vi "UHR-Fleezers Control (fpga) - avogadro 4 - laser switching test.vi"() -> ()   [LabVIEW 2014]
doc: "UHR-Fleezers Instrument Control Code (fpga)"
uses:
  <vilib>/Platform/TimedLoop/XDataNode/timing_clust.ctl
  <vilib>/Platform/TimedLoop/XDataNode/nitl_modes.ctl
  <vilib>/Platform/TimedLoop/XDataNode/wakeup.ctl
  <vilib>/rvi/Emulation/niFpgaGetClockAttributes.vi
  <vilib>/rvi/Emulation/niFpgaSctlEmulationGetInTimedLoop.vi
  <vilib>/rvi/Emulation/niFpgaEmulationReportErrorSimple.vi
  <vilib>/rvi/Emulation/niFpgaProcessEmulError.vi
  <vilib>/rvi/eio/common/nirviEmuTemplateMethod_errors.vi
  <vilib>/rvi/interface/RandomDataEmulation/niFpgaRandomDataHandleErrors.vi
  <vilib>/rvi/Emulation/niFpgaCriticalErrorInLSC.vi
  <vilib>/rvi/Emulation/niFpgaEmulationIsFPGAContextNoSignature.vi
  <vilib>/rvi/errors/niFpgaSetErrorForExecOnDevCompSimple.vi
  <vilib>/rvi/eio/common/nirviEmuReportErrorAndStop.vi
  <vilib>/rvi/DataTransferAndStorage/Container/Common/niFpgaContainerGetUniqueNameForEmu.vi
  <vilib>/rvi/FIFO/Fifo_Resource/nirvififoEmulationSetSize.vi
  <vilib>/rvi/FIFO/Fifo_Resource/nirviFifoEmulationQueueMgr.vi
  <instcachedir>/0/nirviFifoEmulationQueueMgr_E5CAEC123FF24DC58D834DCA3CDAA9B5.lvgen/nirviFifoEmulationQueueMgr_E5CAEC123FF24DC58D834DCA3CDAA9B5_001.vi
  <vilib>/rvi/FIFO/Fifo_Resource/nirvififoEmulationDetermineInputValidOut.vi
  <vilib>/rvi/FIFO/Fifo_Resource/nirvififoEmulationCreateLock.vi
  <vilib>/rvi/FIFO/Fifo_Resource/nirvififoEmulationObtainLock.vi
  <vilib>/rvi/FIFO/Fifo_Resource/nirvififoEmulationReleaseLock.vi
  <vilib>/rvi/occurrence/nirviWaitOnOccurrenceBase.vi
  <vilib>/rvi/errors/nirviReportUnexpectedCaseInternalError.vi
  <vilib>/rvi/errors/nirviReportUnexpectedCaseInternalError (U32).vi
  <vilib>/rvi/DataTransferAndStorage/Container/Common/niFpgaContainerExecOnDevCompGetState.vi
  <vilib>/Utility/error.llb/Clear Errors.vi
  <vilib>/rvi/Memory/Memory_Emulation/niFpgaMemoryEmulationCacheClearOnFirstRun.vi
  <vilib>/rvi/Memory/Memory_Emulation/nirvimemoryEmulationManagerCache_MakeExclusive.vi
  <vilib>/rvi/Memory/Memory_Emulation/niFpgaMemoryEmulationValidateCache.vi
  <vilib>/rvi/Memory/Memory_Emulation/nirvimemoryEmulationManagerCache_InsertValue.vi
  <vilib>/rvi/Memory/Memory_Emulation/nirvimemoryEmulationManagerCache_ReleaseExclusive.vi
  <vilib>/rvi/Memory/Memory_Emulation/nirvimemoryEmulationManagerCache_GetValue.vi
  <vilib>/rvi/Memory/Memory_Emulation/nirvimemoryEmulationManagerCache_SetValue.vi
  <vilib>/rvi/Emulation/niFpgaSctlEmulationResourceMgr.vi
  <vilib>/eio/EIONode/EIONode.xnode
  <vilib>/eio/EIOMethodNode/EIOMethodNode.xnode
  <vilib>/rvi/DataTransferAndStorage/Container/XNode/niFpgaContainer.xnode
  <vilib>/rvi/interface/RandomDataEmulation/nirviRandomDataFpgaReadWriteTemplate.vi
  <vilib>/rvi/FIFO/Fifo_Resource/nirvififoEmulationWrite.vi
  <vilib>/rvi/FIFO/Fifo_Resource/niFpgaFifoEmulationRefIn.vi
  <vilib>/rvi/Memory/Memory_Emulation/niFpgaMemoryEmulationRefIn.vi
  <vilib>/addons/control/pid/fpga.llb/XNode/niFpgaPID.xnode
  <vilib>/Platform/TimedLoop/XDataNode/XDataNode.xnode
  <vilib>/rvi/FIFO/Fifo_Resource/nirvififoEmulationRead.vi
  <vilib>/Platform/TimedLoop/XDataNode/XDNodeRunTimeDep.lvlib
panel:
  in  "BD 1 Delay (ticks)":u8
  out "lifetime (ticks)":u16
  in  "Lifetime to FIFO":bool
  in  "Tab Control":T1(tab)=enum."MCL trap control"
  in  "Set 3":bool
  in  "Set 2":bool=TRUE
  in  "Set 1":bool=TRUE
  in  "Trap Pos to FIFO":bool
  in  "N of AI1 Int Acq Sets":i16=2 min=1 max=3 step=1
  out "AI Late Counter":u8
  in  "ai count":u16=400
  in  "+ phase":bool
  in  "Phase count adjustment":i16
  out "Relative phase":i16
  in  "AI to FIFO":bool
  out "BD1 Frequency Out 1":u64
  out "BD1 Frequency Out 2":u64
  out "Trap Pos FIFO Timeout":u16
  out "Trap AI FIFO Timeout":u16
  in  "Trap FIFO Set Timeout":i32
  in  "Tab Control 2":T2(tab)
  in  "Multiple trap 3 position offset \nfile":bool
  in  "Piezo offset Y points":u64
  in  "Piezo offset X points":u64
  in  "Piezo offset Xmin":u64
  in  "Piezo Offset Ymin":u64
  in  "Piezo Offset Increment":u64
  out "BD1 amplitude 1 out":u16
  out "BD1 amplitude 2 out":u16
  in  "FB output range":cluster{"output low":i16, "output high":i16}={"output low"=0, "output high"=3000}
  in  "FB Gains":T3={"proportional gain (Kc)"=10, "integral gain (Kc*Ts/Ti)"=5, "derivative gain (Kc*Td/Ts)"=0}
  in  "RF synth green feedback max":i16=4000
  in  "RD":bool=TRUE
  in  "Swap F1 and F2":bool
  in  "Cont. Scan":bool
  in  "Abort scan":bool
  in  "Cycles per step":u64
  in  "Scan BD":bool
  in  "Number of scans":u16
  in  "Scan steps":u64
  in  "Scan freq.  increment":i64
  out "Scanning":bool
  in  "Start scan":bool
  in  "OSK Bd 1":bool
  in  "Reset Bd 1":bool
  in  "PMODE":bool=TRUE
  in  "Number Interlace Cycles":u8=2 min=1 max=3
  in  "Interlace Off Parameters":u8=1 min=1 max=3
  in  "Interlace ON/OFF":bool
  out "DIO Relative phase":i16
  in  "Phase count adjustment (DIO)":i16
  in  "+ phase (DIO)":bool
  out "DIO Late Counter":u8
  in  "DIO count 1 (ticks)":u16=400
  in  "DIO count 2 (ticks)":u16=400
  in  "DIO count 3 (ticks)":u16=400
  out "AI2 Y Sum Set 2":i16
  out "AI2 Y Sum Set 1":i16
  in  "FB Setpoint Set 1":i16 min=0 step=1
  in  "FB Reset Set 1":bool
  in  "FB On/Off Set 1":bool
  in  "FB Reset Set 2":bool
  in  "FB On/Off Set 2":bool
  in  "FB Setpoint Set 2":i16 min=0 step=1
  out "Scan I":u64
  in  "Amp switch delay":u8=5
  in  "RF synth bd controls green":bool
  in  "Phase Trap 2":fxp<+,14,14>
  in  "Phase Trap 1":fxp<+,14,14>
  in  "Phase offset method":u8
  in  "BD 2 Amplitude 1":u16
  in  "BD 1 Amplitude 1":u16
  in  "BD 2 Frequency 1":u64
  in  "BD 1 Frequency 1":u64
  in  "BD 2 Amplitude 2":u16
  in  "BD 1 Amplitude 2":u16
  in  "BD 2 Frequency 2":u64
  in  "BD 1 Frequency 2":u64
  in  "BD 2 Amplitude 3":u16
  in  "BD 1 Amplitude 3":u16
  in  "BD 2 Frequency 3":u64
  in  "BD 1 Frequency 3":u64
  in  "BD 2 Delay (Ticks)":u8 caption="Count(Ticks)"
  in  "Next trap write delay (ticks)":u8 caption="Count(Ticks)"
  out "Random phase generated":fxp<+,14,14>
  in  "RF phase reset before cycles":bool
  in  "Trap 1 osc enable":bool
  in  "N trap osc periods":i16
  in  "Trap osc period (pts)":i16
  in  "Osc traps":bool
  in  "Initiate trap osc":bool
  in  "Ready Write":bool
  in  "Data":i64
  in  "Address 2":u32
  in  "Osc trap cont.":bool
  in  "Trap 2 osc enable":bool
  out "Piezo X out":i16
  out "Piezo Y out":i16
  in  "Piezo Trap ON/Off (AO3)":i16
  in  "Piezo Trap X (AO5)":i16
  in  "Piezo Trap Y (AO4)":i16
  in  "FB Min frequency":u64
  in  "FB Max Frequency":u64
  in  "Dynamic Force FB (Ronen)":bool
  in  "Trap pos. FB Range":T4={"FB2 output low"=-1.0, "FB2 output high"=0.999969482421875}
  in  "Trap Pos. FB Gains":T5={"proportional gain (Kc)"=0.999969482421875, "integral gain (Kc*Ts/Ti)"=0.999969482421875, "derivative gain (Kc*Td/Ts)"=0.0}
  in  "B factor":fxp<+/-,32,16>
  in  "Negate Diff?":bool
  in  "Diff FB Measurement?":bool
  in  "FB Trig Integrate":u32=1
  out "TTrig?":bool
  in  "TTrig Negate Pos":bool=TRUE
  out "Trap Pos FB Int Signal":fxp<+/-,24,9> format="%.18g"
  out "Trap Pos FB Int-Norm Signal":fxp<+/-,16,1> format="%.16g"
  in  "FPGA TTrig Thresh":i64
  in  "FPGA Trap Trig":bool
  out "Trap Pos FB Action":i64
  in  "Trap Pos. FB Offset Factor":i64
  in  "Trap Pos. FB Mult Factor":i64=2
  in  "Trap Pos. FB Reset":bool
  in  "Trap Pos FB Monitor T1 or T2":bool
  in  "AI1 X Scale":u16
  in  "Trap Pos FB Int Count":u16=100
  in  "Trap Pos FB Negate Action":bool
  out "AI1 X Set 2":fxp<+/-,16,1>
  out "AI1 X Set 1":fxp<+/-,16,1>
  in  "Trap Pos. FB SP":fxp<+/-,16,1>
  in  "Force feedback":bool
  out "TTrig Sig":i64
  out "TTrig Fin Thresh":i64
  in  "ScanTrap 3 or Fl-laser":bool
  in  "1D or 2D Scan?":bool
  in  "Abort scan (MCL)":bool
  in  "MCL Scan Axis":bool
  in  "Cont. Scan (MCL)":bool
  out "Scan I (MCL)":u64
  in  "Number of scans (MCL)":u16
  out "Scanning MCL":bool
  in  "Scan steps (MCL)":u64
  in  "Cycles per step (MCL)":u64
  in  "Scan freq.  increment (MCL)":i16
  in  "Start scan (MCL)":bool
  in  "AO2 (X)":i16
  in  "AO1 (Y)":i16
  out "MCL Late Counter":u8
  in  "MCL count":u32=800
  out "MCL Relative Phase":i16
  in  "Phase count adjustment (MCL)":i16
  in  "+ phase (MCL)":bool
  in  "Lifetime events to read blue":u16=100
  in  "Lifetime read blue fifo":bool
  out "lifetime events in fifo":u16
  out "APD2 int gate":bool
  out "APD3 out state":bool
  in  "APD Gate Operating Mode":u8 max=2 step=1
  in  "Invert APD Gate":bool
  in  "APD Gate OFF Count":u16=100
  in  "APD Gate ON Count":u16=300
  out "APD 1 Gate Late Counter":u8
  out "APD 1 Gate Relative Phase":i16
  in  "Phase count adjustment (APD 1 Gate)":i16
  in  "+ phase (APD 1 Gate)":bool
  out "APD 2 Counts 0":u32
  out "APD 2 Counts 1":u32
  out "APD 1 Counts 0":u32
  out "APD 1 Counts 1":u32
  out "APD1 out state":bool
  in  "APD AO scale factor":i16=1
  in  "APD to FIFO":bool
  in  "APD Acq Rate Count":u32=20000000
  out "APD Acq Late Counter":u8
  out "APD Acq Relative Phase":i16
  in  "Phase Count Adjustment (APD Acq)":i16
  in  "+ phase (APD Acq)":bool
  in  "Phase count adjustment (APD 2 Gate)":i16
  out "APD 2 Gate Late Counter":u8
  out "APD 2 Gate Relative Phase":i16
  in  "+ phase (APD 2 Gate)":bool
  out "APD2 out state":bool
  out "APD 3 Counts 0":u32
  out "APD 3 Counts 1":u32
  out "APD 3 Gate Late Counter":u8
  in  "Phase count adjustment (APD 3 Gate)":i16
  out "APD 3 Gate Relative Phase":i16
  in  "+ phase (APD 3 Gate)":bool
  out "APD1 int gate":bool
  out "APD3 int gate":bool
  in  "Lifetime timeout APD1":u16=200
  in  "Laser choice 2":u8=100
  in  "Laser choice 1":u8=100
  in  "Laser choice 0":u8=100
  in  "FL interlace OFF count 2":u16=100
  in  "FL interlace OFF count 1":u16=100
  in  "FL interlace ON count 2":u16=300
  in  "Fl interlace ON count 1":u16=300
  in  "D3 2":i16
  in  "I3 2":i16=5
  in  "P3 2":i16=10
  in  "Green FB Setpoint 2":i16=250 min=0 step=1
  in  "Green FB Reset 2":bool
  in  "D3":i16
  in  "I3":i16=5
  in  "P3":i16=10
  in  "Green Filter Flipper":bool
  in  "Green FB Count":u16=1200
  out "Green Late Counter":u8
  out "Green FB Relative Phase":i16
  in  "Phase count adjustment (Green FB)":i16=10
  in  "+ phase (Green FB)":bool
  out "Green FB Sum":i16
  in  "Green int current ON count adj":u16=150
  in  "Current Out":u16=30000
  in  "Green FB On/Off":bool
  in  "Green FB Setpoint":i16=250 min=0 step=1
  in  "Green FB Reset":bool
  in  "Operating Mode 2":u8=2 max=2 step=1
  in  "Invert GI 2":bool
  in  "Green interlace OFF count 2":u16=900
  in  "Green interlace ON count 2":u16=300
  out "GI Late Counter 2":u8
  out "GI Relative phase 2":i16
  in  "Phase count adjustment (GI) 2":i16=20
  in  "+ phase (GI) 2":bool
  in  "FL interlace OFF count 0":u16=100
  out "GI Relative phase":i16
  in  "Phase count adjustment (GI)":i16
  in  "+ phase (GI)":bool
  in  "FL interlace ON count 0":u16=300
  out "GI Late Counter":u8
  in  "Invert GI":bool
  in  "Operating Mode":u8 max=2 step=1
  out "green FB running":bool
  in  "+ phase (RI)":bool
  out "RI Relative phase":i16
  out "RI Late Counter":u8
  in  "Red interlace ON count":u16=300
  in  "Red interlace OFF count":u16=100
  in  "Invert RI":bool
  in  "Red Laser Operating Mode":u8 max=2 step=1
  in  "Phase count adjustment (RI)":i16
  out "Red FB Intensity":i16
  in  "RI Current Out":u16=30000
  in  "Red FB On/Off":bool
  in  "D4":i16
  in  "I4":i16=5
  in  "P4":i16=10
  in  "Red FB Setpoint":i16=250 min=0 step=1
  in  "Red FB Reset":bool
  in  "RI Operating Mode 2":u8=2 max=2 step=1
  in  "Invert RI 2":bool
  in  "Phase count adjustment (BI AO)":i16=20
  in  "Blue current ON count adj (AO)":u16=150
  in  "BI Current Out":i16=30000
  in  "Blue FB On/Off":bool
  in  "D5":i16
  in  "I5":i16=5
  in  "P5":i16=10
  in  "Blue FB Setpoint":i16=250 min=0 step=1
  in  "Blue FB Reset":bool
  in  "BI Operating Mode (AO)":u8=2 max=2 step=1
  in  "Invert BI (AO)":bool
  in  "Blue OFF count (AO)":u16=900
  in  "Blue ON count (AO)":u16=300
  out "BI Late Counter (AO)":u8
  out "BI Relative phase (AO)":i16
  in  "+ phase (BI AO)":bool
  in  "Phase count adjustment (BI D)":i16
  in  "Blue Laser Operating Mode (D)":u8 max=2 step=1
  in  "Invert BI (D)":bool
  in  "Blue interlace OFF count (D)":u16=100
  in  "Blue interlace ON count (D)":u16=300
  out "Blue Late Counter (D)":u8
  out "BI Relative phase (D)":i16
  in  "+ phase (BI D)":bool
  out "Blue Intensity":i16
  in  "Invert EMCCD Gate":bool
  in  "EMCCD Gate ON count":u16=300
  in  "EMCCD Gate OFF count":u16=100
  out "EMCCD Late counter":u8
  out "EMCCD relative phase":i16
  in  "+ phase (EMCCD Gate)":bool
  in  "EMCCD Gate Operating Mode":u8 max=2 step=1
  in  "Phase Count Adjustment EMCCD Gate":i16
  # "Raster Scan AOD"
  # "1 (X)"
  # "2 (Y)"
  # "IR Intensity Feedback (RF BD 1)"
  # "FB Gains Set 1"
  # "FB output range 1"
  # "IR Intensity Feedback (RF BD 2) -\nonly when using BD 2 for green laser AOM (not trap Y)"
  # "Keep below 4096 (12 bits) to stay within range of RF board. Going over doesn't saturate, it truncates higher bits."
  # "RF phase offset control"
  # "Methods are:\n0 - Default, do nothing at all (no phase offset writes)\n1 - Manual phase adjustment\n2 - Cycle the phase adjustment using the input phase numbers as increment values for each cycle"
  # "False is usual, True is external loop method"
  # "Parameters if using the external RF switching loop"
  # "Parameters if using the usual internal RF switching method"
  # "FB Triggering Excitation Laser"
  # "Trap Pos. FB Gains"
  # "Trap Pos. FB Range"
  # "AO1 (Y)"
  # "2D"
  # "Trap 3"
  # "1D"
  # "AO2 (X)"
  # "Fl Laser"
  # "APD AO for aligning"
  # "Detection Loop"
  # "Green fluorescent laser digital gate interlacing loop"
  # "0 Forced ON\n1 Forced OFF\n2 Interlacing"
  # "ALEX settings:"
  # "Controls for usual IA ME controls green AOM"
  # "Controls for RF synth board controls green AOM"
  # "Green FB Gains"
  # "Red fluorescent laser digital gate interlacing loop"
  # "Detection Loop"
  # "0 Forced ON\n1 Forced OFF\n2 Interlacing"
  # "Analog/FB Control Loop\n(Disabled)"
  # "Digital Control Loop"
  # "Blue laser intensity reading"
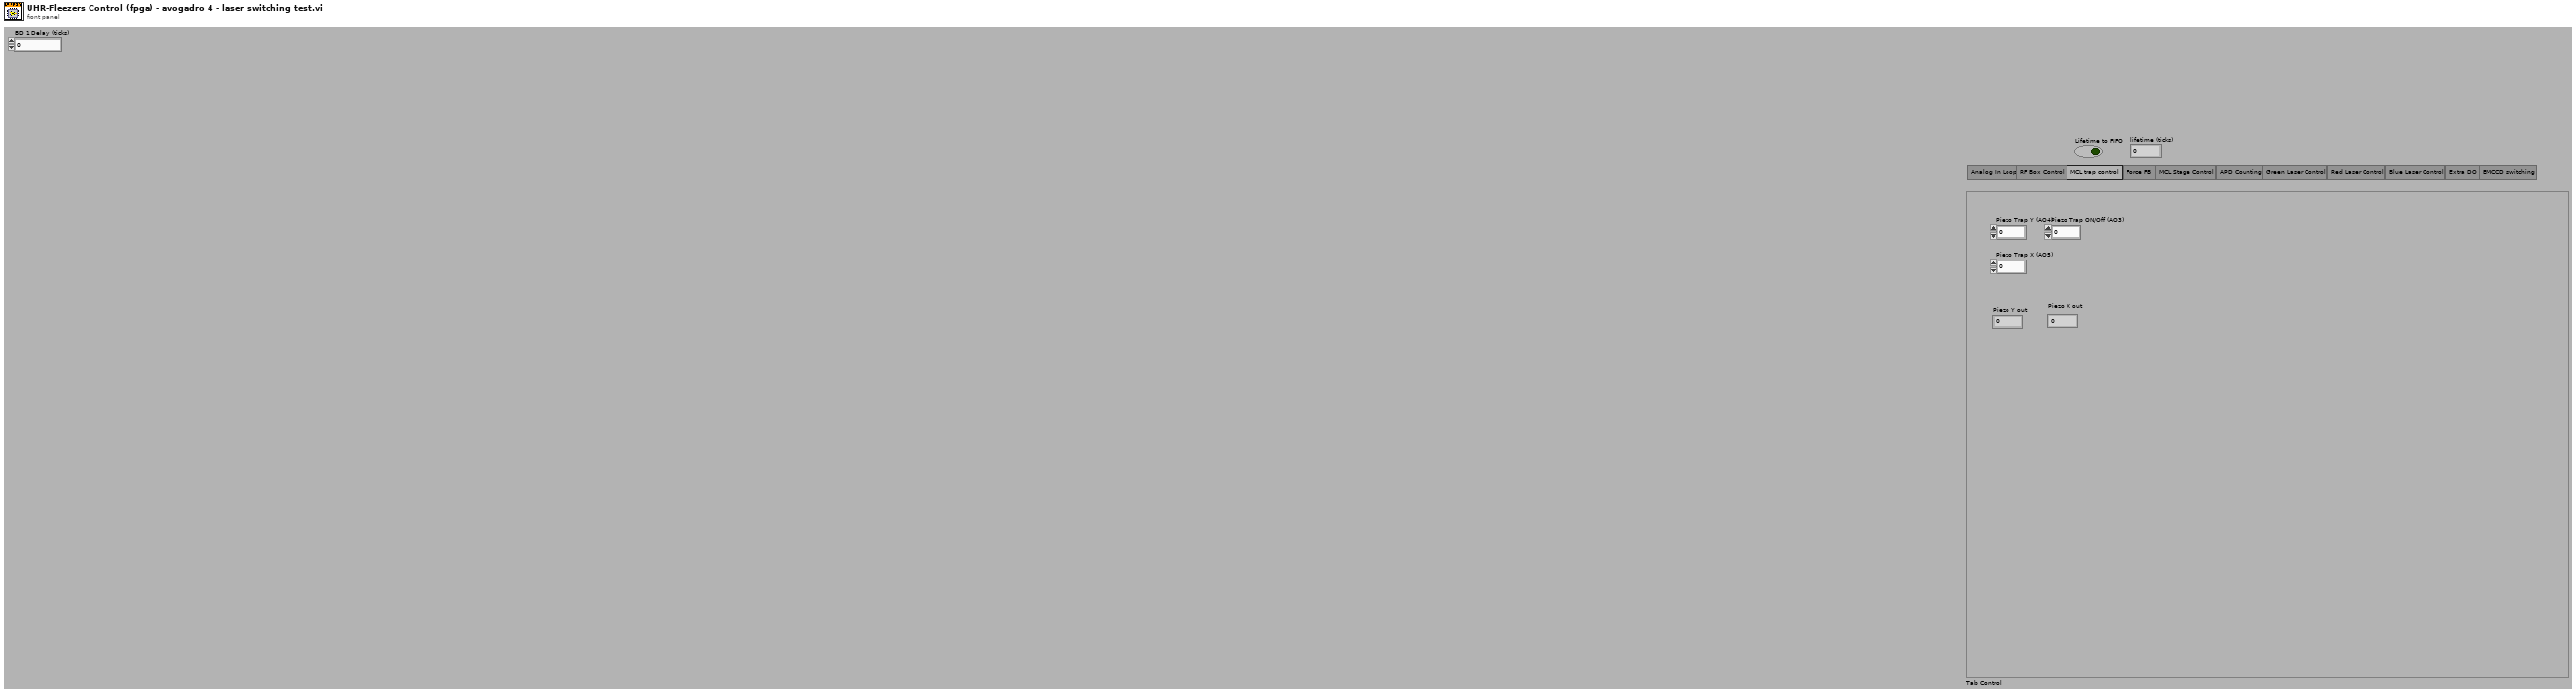
[diagram p1: front panel]
types:
  T1 = enum32{"Analog In Loop", "RF Box Control", "MCL trap control", "Force FB", "MCL Stage Control", "APD Counting", "Green Laser Control", "Red Laser Control", "Blue Laser Control", "Extra DO", "EMCCD switching"}
  T2 = enum32{"Controls", "Interlacing Frequency and Amplitude Values", "Oscillate trap from memory"}
  T3 = cluster{"proportional gain (Kc)":i16, "integral gain (Kc*Ts/Ti)":i16, "derivative gain (Kc*Td/Ts)":i16}
  T4 = cluster{"FB2 output low":fxp<+/-,16,1>, "FB2 output high":fxp<+/-,16,1>}
  T5 = cluster{"proportional gain (Kc)":fxp<+/-,16,1>, "integral gain (Kc*Ts/Ti)":fxp<+/-,16,1>, "derivative gain (Kc*Td/Ts)":fxp<+/-,16,1>}
  T6 = typedef "XDNodeRunTimeDep.lvlib/timing_clust.ctl" = cluster{"Expected End [f-1]":u64, "Actual End [f-1]":u64, "Finished Late? [f-1]":bool, "Expected End [i-1]":u64, "Actual End [i-1]":u64, "Finished Late? [i-1]":bool, "Expected Start [i]":u64, "Actual Start [i]":u64, "Expected Start [f]":u64, "Actual Start [f]":u64, "Source Name":string, "Structure Name":string, "Period":i64, "Deadline":i64, "Offset":i64, "Start":i64, "Priority":i32, "Timeout":i32, "Mode":T7, "Wakeup Reason":T8, "Error":errorcluster, "Source Type":string, "Secondary Source Type":string, "Global End Time":u64, "Global Start Time":u64, "Frame Duration":u64, "Iteration Duration":u64, "Assigned CPU":i32, "I/O Scan Engine Mode":u32}
  T7 = typedef "XDNodeRunTimeDep.lvlib/nitl_modes.ctl" = enum32{"No Change", "Process missed periods, maintain original phase", "Discard missed periods, maintain original phase", "Process missed periods, ignore original phase", "Discard missed periods, ignore original phase"}
  T8 = typedef "XDNodeRunTimeDep.lvlib/wakeup.ctl" = enum32{"Normal", "Aborted", "Asynchronous wakeup", "Timing source error", "Timed loop error", "Timeout"}
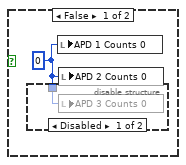
[diagram p4: hidden frame]
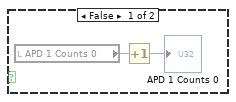
[diagram p9: hidden frame]
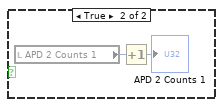
[diagram p11: hidden frame]
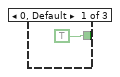
[diagram p13: hidden frame]
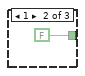
[diagram p14: hidden frame]
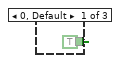
[diagram p15: hidden frame]
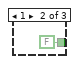
[diagram p16: hidden frame]
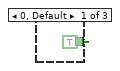
[diagram p18: hidden frame]
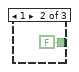
[diagram p19: hidden frame]
diagram:
  w10 = i16 0
  w14 = FALSE
  # "EMCCD gating"
  # "BD2 amp"
  # "BD1 amp"
  # "BD2 amp"
  # "BD1 amp"
  # "timing array current index"
  # "timing array"
  # "timing counter (phase adjusted here)"
  # "late counter"
  n1 = disable-structure shown="Disabled" {
    frame Disabled {
      w15 = i16 2 items=["UnSet Ready", "ReadWrite", "Wait Ready"]
      n2 = while "Handshake memory transfer for trap oscillation sin wave data" {
        shift-right: [w17] -> _
        shift-left: w15 -> [w18]
        stop <- FALSE stop-if-true
        # "Write"
        n3 = case shown="1" w18 {
          tunnel: [w21 w26 w27] -> w17
          frame 3, Default {
            w19 = i16 2 items=["UnSet Ready", "ReadWrite", "Wait Ready"]
            w20 = i16 1 items=["UnSet Ready", "ReadWrite", "Wait Ready"]
            n4 = Select(t=w20, s="Ready Write", f=w19) -> (s? t:f=w21:i16)
          }
          frame 1 {
            w26 = i16 0 items=["UnSet Ready", "ReadWrite", "Wait Ready"]
            n5 = xnode ("Memory Write")("Address"="Address 2", "Data"="Data", "Memory In"=refnum<k21> "Trap osc memory") -> ()  [unwired: 1 out]
          }
          frame 0 {
            w27 = i16 2 items=["UnSet Ready", "ReadWrite", "Wait Ready"]
            n6 = local write "Ready Write"(FALSE ("Ready Read")) -> ()
          }
        }
      }
    }
    frame Enabled {
    }
  }
  n7 = flat-sequence "FPGA initialization to do before running any of the loops" {
    tunnel: [u16 0 ("DIO count 3 (ticks)")] -> w2
    tunnel: [w36] -> _
    frame #0 {
      # "UDCLK out enable and set low"
      # "WR"
      # "BD 2"
      # "BD 1"
      # "With the RF synth board initialization now done in a separate fpga vi, now when this vi is started, board is already configured and is ready for interlacing. Just need to set WR high and enabled UDCLK as write and set to low.\nbefore setting data and address bits."
      # "Start up expansion chassis early\nto avoid delays later"
      # "Set data and address values to something safe (a correct setting) so any initial WR and udclk flipping doesn't have a chance to mess anything up. Safe would be setting an unused data entry:"
      n8 = xnode "FPGA I/O Method Node"("Enable"=TRUE) -> ("FPGA I/O Out"=w30:refnum<k21>)  [unwired: 1 in]
      n9 = xnode "FPGA I/O Method Node"("Enable"=TRUE) -> ("FPGA I/O Out"=w33:refnum<k21>)  [unwired: 1 in]
      n10 = xnode "FPGA I/O Node"("Chassis2/Mod1/AO0"=u16 0 ("Chassis2/Mod4/AO0")) -> ("Chassis2/Mod2/AI0"=w36:i16)  [unwired: 2 in, 2 out]
      n11 = xnode "FPGA I/O Node"("Connector1/DIO15"=TRUE) -> ()  [unwired: 1 in, 1 out]
      n12 = xnode "FPGA I/O Node"("I/O Item"=FALSE ("Connector1/DIO30"), "FPGA I/O In"=w30) -> ()  [unwired: 1 out]
      n13 = xnode "FPGA I/O Node"("I/O Item"=FALSE ("Connector1/DIO30"), "FPGA I/O In"=w33) -> ()  [unwired: 1 out]
      n14 = xnode "FPGA I/O Node"("Connector1/DIO0"=FALSE, "Connector1/DIO1"=FALSE, "Connector1/DIO2"=FALSE, "Connector1/DIO3"=FALSE, "Connector1/DIO4"=FALSE, "Connector1/DIO5"=FALSE, "Connector1/DIO6"=FALSE, "Connector1/DIO7"=FALSE, "Connector1/DIO8"=FALSE, "Connector1/DIO9"=FALSE, "Connector1/DIO10"=FALSE, "Connector1/DIO11"=FALSE, "Connector1/DIO12"=FALSE, "Connector1/DIO13"=FALSE, "Connector1/DIO20"=FALSE, "Connector1/DIO21"=FALSE, "Connector1/DIO22"=FALSE, "Connector1/DIO23"=FALSE, "Connector1/DIO24"=FALSE, "Connector1/DIO25"=FALSE, "Connector1/DIO26"=FALSE, "Connector1/DIO27"=FALSE, "Connector1/DIO14"=FALSE) -> ()  [unwired: 23 in, 23 out]
    }
  }
  n15 = node-c288() -> (w5:T6)  [unwired: 1 in]
  n16 = timed-loop "RF box board DIO control: control bits" {
    timing: w5 -> [_]
    timing-out: [_] -> w4
    tunnel: [w64] -> _
    tunnel: w2 -> [w64]
    stop <- FALSE stop-if-true
    n17 = xnode "FPGA I/O Node"("Connector1/DIO16"="RD", "Connector1/DIO17"="PMODE", "Connector1/DIO18"="OSK Bd 1", "Connector1/DIO19"="Reset Bd 1", "Connector0/DIO3"="Green Filter Flipper") -> ()  [unwired: 5 in, 5 out]
  }
  n18 = node-c288(w4) -> ()
  n19 = local read "AO1 (Y)"() -> (w12:i16)
  n20 = local read "AO2 (X)"() -> (w11:i16)
  n21 = To Unsigned Long Integer(number=w2) -> (unsigned 32bit integer=w1:u32)
  n22 = disable-structure shown="Disabled" {
    disable-tunnel: w2 -> [w72 _]
    disable-tunnel: [w71 _] -> w3
    frame Disabled {
      w71 = FALSE
      n23 = while "APD 1 Gating" {
        shift-right: [w127] -> _
        shift-left: w72 -> [w132]
        shift-right: [w126] -> _
        shift-left: w71 -> [w124]
        stop <- FALSE stop-if-true
        n24 = flat-sequence {
          tunnel: w132 -> [w135]
          tunnel: [w136] -> w130
          tunnel: [w135] -> w128
          tunnel: [w134] -> w125
          tunnel: w124 -> [w134]
          tunnel: [w139] -> w131
          tunnel: w130 -> [w139]
          tunnel: [w138] -> w129
          tunnel: w128 -> [w138]
          tunnel: w125 -> [w137]
          tunnel: [w157] -> w127
          tunnel: w131 -> [w171]
          tunnel: w129 -> [w168]
          tunnel: [w140] -> w126
          frame #0 {
            n25 = call "Loop Timer7"("Count(Ticks)"=w135) -> ("Tick Count(Ticks)"=w136:u16)
          }
          frame #1 {
            # "Signal maybe then sent through \na transistor before APD"
            n26 = xnode "FPGA I/O Node"("Connector0/DIO0"=w137) -> ()  [unwired: 1 in, 1 out]
            "APD1 int gate" <- w137
          }
          frame #2 {
            n27 = feedback #1(TRUE) -> (w163:bool)
            n28 = feedback-in #2(w171) -> ()
            n29 = feedback #2(w171) -> (w170:u16)
            n30 = Not(x=w163) -> (.not. x?=w160:bool)
            n31 = feedback-in #1(w160) -> ()
            n32 = Subtract(x=w171, y=w170) -> (x-y=w169:u16)
            n33 = Select(t="APD Gate ON Count", s=w160, f="APD Gate OFF Count") -> (s? t:f=w165:u16)
            n34 = Subtract(x=w169, y=w168) -> (x-y=w145:u16)
            n35 = Subtract(x=w165, y=w145) -> (x-y=w156:u16)
            n36 = Number To Boolean Array(number=w145) -> (Boolean array=w146:bool[])
            n37 = Or Array Elements(Boolean array=w146) -> (logical OR=w144:bool)
            n38 = Boolean To (0,1)(Boolean="+ phase (APD 1 Gate)") -> (0, 1=w154:i16)
            n39 = Boolean To (0,1)(Boolean=w144) -> (0, 1=w151:i16)
            n40 = Multiply(x=w154, y="Phase count adjustment (APD 1 Gate)") -> (x*y=w152:i16)
            n41 = To Unsigned Byte Integer(number=w151) -> (unsigned 8bit integer=w148:u8)
            n42 = Add(x=w156, y=w152) -> (x+y=w157:u16)
            n43 = feedback #3(i16 0) -> (w159:i16)
            n44 = Subtract(x=w159, y=w152) -> (x-y=w158:i16)
            "APD 1 Gate Relative Phase" <- w158
            n45 = feedback-in #3(w158) -> ()
            n46 = feedback #4(u8 0) -> (w149:u8)
            n47 = Add(x=w148, y=w149) -> (x+y=w147:u8)
            "APD 1 Gate Late Counter" <- w147
            n48 = feedback-in #4(w147) -> ()
            n49 = case shown="2" "APD Gate Operating Mode" {
              tunnel: [TRUE FALSE w174] -> w141
              tunnel: w163 -> [_ _ w174]
              frame 0, Default {
              }
              frame 1 {
              }
              frame 2 {
              }
            }
            n50 = Not(x=w141) -> (.not. x?=w142:bool)
            n51 = Select(t=w142, s="Invert APD Gate", f=w141) -> (s? t:f=w140:bool)
          }
        }
      }
      n52 = while "APD 2 Gating" {
        shift-right: [w76] -> _
        shift-left: w72 -> [w81]
        shift-right: [w75] -> _
        shift-left: w71 -> [w73]
        stop <- FALSE stop-if-true
        n53 = flat-sequence {
          tunnel: w81 -> [w84]
          tunnel: [w85] -> w79
          tunnel: [w84] -> w77
          tunnel: [w83] -> w74
          tunnel: w73 -> [w83]
          tunnel: [w88] -> w80
          tunnel: w79 -> [w88]
          tunnel: [w87] -> w78
          tunnel: w77 -> [w87]
          tunnel: w74 -> [w86]
          tunnel: [w110] -> w76
          tunnel: w80 -> [w120]
          tunnel: w78 -> [w118]
          tunnel: [w89] -> w75
          frame #0 {
            n54 = call "Loop Timer8"("Count(Ticks)"=w84) -> ("Tick Count(Ticks)"=w85:u16)
          }
          frame #1 {
            # "Signal maybe then sent through \na transistor before APD"
            n55 = xnode "FPGA I/O Node"("Connector0/DIO1"=w86) -> ()  [unwired: 1 in, 1 out]
            "APD2 int gate" <- w86
          }
          frame #2 {
            n56 = local read "APD Gate ON Count"() -> (w103:u16)
            n57 = local read "APD Gate OFF Count"() -> (w102:u16)
            n58 = feedback #5(TRUE) -> (w115:bool)
            n59 = feedback-in #6(w120) -> ()
            n60 = feedback #6(w120) -> (w104:u16)
            n61 = Not(x=w115) -> (.not. x?=w113:bool)
            n62 = feedback-in #5(w113) -> ()
            n63 = Subtract(x=w120, y=w104) -> (x-y=w119:u16)
            n64 = Select(t=w103, s=w113, f=w102) -> (s? t:f=w117:u16)
            n65 = Subtract(x=w119, y=w118) -> (x-y=w95:u16)
            n66 = Subtract(x=w117, y=w95) -> (x-y=w109:u16)
            n67 = Number To Boolean Array(number=w95) -> (Boolean array=w94:bool[])
            n68 = Or Array Elements(Boolean array=w94) -> (logical OR=w93:bool)
            n69 = Boolean To (0,1)(Boolean="+ phase (APD 2 Gate)") -> (0, 1=w107:i16)
            n70 = Multiply(x=w107, y="Phase count adjustment (APD 2 Gate)") -> (x*y=w105:i16)
            n71 = Boolean To (0,1)(Boolean=w93) -> (0, 1=w100:i16)
            n72 = Add(x=w109, y=w105) -> (x+y=w110:u16)
            n73 = To Unsigned Byte Integer(number=w100) -> (unsigned 8bit integer=w97:u8)
            n74 = feedback #7(i16 0) -> (w112:i16)
            n75 = Subtract(x=w112, y=w105) -> (x-y=w111:i16)
            "APD 2 Gate Relative Phase" <- w111
            n76 = feedback-in #7(w111) -> ()
            n77 = feedback #8(u8 0) -> (w98:u8)
            n78 = Add(x=w97, y=w98) -> (x+y=w96:u8)
            "APD 2 Gate Late Counter" <- w96
            n79 = feedback-in #8(w96) -> ()
            n80 = local read "APD Gate Operating Mode"() -> (w101:u8)
            n81 = case shown="2" w101 {
              tunnel: [TRUE FALSE w123] -> w90
              tunnel: w115 -> [_ _ w123]
              frame 0, Default {
              }
              frame 1 {
              }
              frame 2 {
              }
            }
            n82 = local read "Invert APD Gate"() -> (w92:bool)
            n83 = Not(x=w90) -> (.not. x?=w91:bool)
            n84 = Select(t=w91, s=w92, f=w90) -> (s? t:f=w89:bool)
          }
        }
      }
    }
    frame Enabled {
    }
  }
  n85 = disable-structure shown="Disabled" {
    disable-tunnel: w2 -> [w175 _]
    frame Disabled {
      n86 = while "Excitation laser intensity feedback measurement (all lasers)" {
        shift-right: [w176] -> _
        shift-left: w175 -> [w181]
        stop <- FALSE stop-if-true
        n87 = flat-sequence {
          tunnel: w181 -> [w183]
          tunnel: [w184] -> w179
          tunnel: [w183] -> w177
          tunnel: [w190] -> w180
          tunnel: w179 -> [w190]
          tunnel: [w189] -> w178
          tunnel: w177 -> [w189]
          tunnel: [w202] -> w176
          tunnel: w180 -> [w213]
          tunnel: w178 -> [w210]
          frame #0 {
            n88 = call "Loop Timer9"("Count(Ticks)"=w183) -> ("Tick Count(Ticks)"=w184:u16)
          }
          frame #1 {
            # "Design note:\n\nAll lasers need to be measured at the same \ntime because the AI expansion module\ncannot independently time the measurements\nwithin our requirements: there is dead time.\n\nThis probably wouldn't be an issue with the built\nin AI on the fpga board itself."
            n89 = xnode "FPGA I/O Node"("Connector1/DIO35"=TRUE) -> ("Chassis2/Mod1/AI2"=→"Blue Intensity", "Chassis2/Mod1/AI1"=→"Red FB Intensity", "Chassis2/Mod1/AI0"=→"Green FB Sum")  [unwired: 4 in, 4 out]
          }
          frame #2 {
            n90 = feedback-in #9(w213) -> ()
            n91 = feedback #9(w213) -> (w212:u16)
            n92 = Subtract(x=w213, y=w212) -> (x-y=w211:u16)
            n93 = xnode "FPGA I/O Node"("Connector1/DIO35"=FALSE) -> ()  [unwired: 1 in, 1 out]
            n94 = Subtract(x=w211, y=w210) -> (x-y=w192:u16)
            n95 = Subtract(x="Green FB Count", y=w192) -> (x-y=w206:u16)
            n96 = Number To Boolean Array(number=w192) -> (Boolean array=w193:bool[])
            n97 = Or Array Elements(Boolean array=w193) -> (logical OR=w191:bool)
            n98 = Boolean To (0,1)(Boolean="+ phase (Green FB)") -> (0, 1=w204:i16)
            n99 = Boolean To (0,1)(Boolean=w191) -> (0, 1=w198:i16)
            n100 = Multiply(x=w204, y="Phase count adjustment (Green FB)") -> (x*y=w199:i16)
            n101 = Add(x=w206, y=w199) -> (x+y=w202:u16)
            n102 = To Unsigned Byte Integer(number=w198) -> (unsigned 8bit integer=w195:u8)
            n103 = feedback #10(i16 0) -> (w201:i16)
            n104 = Subtract(x=w201, y=w199) -> (x-y=w200:i16)
            "Green FB Relative Phase" <- w200
            n105 = feedback-in #10(w200) -> ()
            n106 = feedback #11(u8 0) -> (w196:u8)
            n107 = Add(x=w195, y=w196) -> (x+y=w194:u8)
            "Green Late Counter" <- w194
            n108 = feedback-in #11(w194) -> ()
          }
        }
      }
    }
    frame Enabled {
    }
  }
  n109 = disable-structure shown="Disabled" {
    disable-tunnel: w2 -> [w214 _]
    frame Disabled {
      n110 = while "APD 2 Counter" {
        tunnel: w214 -> [_]
        stop <- FALSE stop-if-true
        n111 = flat-sequence {
          frame #0 {
            n112 = xnode "FPGA I/O Method Node"("FPGA I/O In"=refnum<k21> "Connector0/DIO8" ("APD 2 DO"), "Timeout"=-1) -> ()  [unwired: 2 out]
          }
          frame #1 {
            n113 = local read "APD2 int gate"() -> (w227:bool)
            n114 = case shown="True" w227 {
              frame False {
              }
              frame True {
                n115 = local read "APD2 out state"() -> (w228:bool)
                n116 = case shown="False" w228 {
                  frame False {
                    n117 = local read "APD 2 Counts 0"() -> (w230:u32)
                    n118 = Increment(x=w230) -> (x+1=→"APD 2 Counts 0":u32)
                  }
                  frame True {
                    n119 = local read "APD 2 Counts 1"() -> (w232:u32)
                    n120 = Increment(x=w232) -> (x+1=→"APD 2 Counts 1":u32)
                  }
                }
              }
            }
          }
        }
      }
      n121 = while "APD 1 Counter" {
        tunnel: w214 -> [_]
        stop <- FALSE stop-if-true
        n122 = flat-sequence {
          frame #0 {
            n123 = xnode "FPGA I/O Method Node"("FPGA I/O In"=refnum<k21> "Connector0/DIO4" ("APD 1 DO"), "Timeout"=-1) -> ()  [unwired: 2 out]
          }
          frame #1 {
            n124 = local read "APD1 int gate"() -> (w218:bool)
            n125 = case shown="True" w218 {
              frame False {
              }
              frame True {
                n126 = local read "APD1 out state"() -> (w219:bool)
                n127 = case shown="True" w219 {
                  frame False {
                    n128 = local read "APD 1 Counts 0"() -> (w221:u32)
                    n129 = Increment(x=w221) -> (x+1=→"APD 1 Counts 0":u32)
                  }
                  frame True {
                    n130 = local read "APD 1 Counts 1"() -> (w223:u32)
                    n131 = Increment(x=w223) -> (x+1=→"APD 1 Counts 1":u32)
                  }
                }
              }
            }
          }
        }
      }
    }
    frame Enabled {
    }
  }
  n132 = disable-structure shown="Disabled" {
    disable-tunnel: w2 -> [w233 _]
    frame Disabled {
      w234 = u16 0
      n133 = while "Green and red fluorescent laser interlacing (Current AO to IA 532 nm AOM ME amp)." {
        shift-right: [w314] -> _
        shift-left: w233 -> [w317]
        shift-right: [w311] -> _
        shift-left: w234 -> [w309]
        shift-right: [w308] -> _
        shift-left: w234 -> [w307]
        stop <- FALSE stop-if-true
        n134 = flat-sequence {
          tunnel: w317 -> [w321]
          tunnel: [w322] -> w316
          tunnel: [w321] -> w315
          tunnel: [w320] -> w310
          tunnel: w309 -> [w320]
          tunnel: w307 -> [w319]
          tunnel: [w319] -> w306
          tunnel: [w326] -> w313
          tunnel: w316 -> [w326]
          tunnel: [w325] -> w312
          tunnel: w315 -> [w325]
          tunnel: w310 -> [w324]
          tunnel: w306 -> [w323]
          tunnel: [w354] -> w314
          tunnel: [w370] -> w311
          tunnel: w313 -> [w381]
          tunnel: w312 -> [w378]
          tunnel: [w339] -> w308
          frame #0 {
            n135 = call "Loop Timer10"("Count(Ticks)"=w321) -> ("Tick Count(Ticks)"=w322:u16)
          }
          frame #1 {
            n136 = xnode "FPGA I/O Node"("Chassis2/Mod4/AO0"=w324, "Chassis2/Mod4/AO1"=w323) -> ()  [unwired: 2 in, 2 out]
          }
          frame #2 {
            # "IF RF synth BD does green, never run FB"
            # "ALEX variable is used by APD acquisition loop\nto turn lasers ON/OFF."
            # "Design note:\n\nThese two laser controls are in the same loop\nbecause the expansion current AI cannot separately\ntime the outputs fast enough for us.  Apparently\nit is because of communication time between the\nexpansion card and the fpga.\n\nSo the two analog control signals have the same timing\nand profile, but independent amplitudes to independently\ncontrol the intensity and feedback for each laser."
            n137 = feedback #12(TRUE) -> (w336:bool)
            n138 = Not(x=w336) -> (.not. x?=w337:bool)
            n139 = feedback-in #12(w337) -> ()
            n140 = Subtract(x="Green interlace OFF count 2", y="Green int current ON count adj") -> (x-y=w363:u16)
            n141 = feedback-in #13(w381) -> ()
            n142 = feedback #13(w381) -> (w380:u16)
            n143 = Add(x="Green int current ON count adj", y="Green interlace ON count 2") -> (x+y=w364:u16)
            n144 = Subtract(x=w381, y=w380) -> (x-y=w379:u16)
            n145 = Select(t=w364, s=w337, f=w363) -> (s? t:f=w375:u16)
            n146 = Subtract(x=w379, y=w378) -> (x-y=w347:u16)
            n147 = case shown="2" "RI Operating Mode 2" {
              tunnel: [TRUE FALSE w387] -> w332
              tunnel: w336 -> [_ _ w384]
              frame 0, Default {
              }
              frame 1 {
              }
              frame 2 {
                n148 = Not(x=w384) -> (.not. x?=w386:bool)
                n149 = Select(t=w386, s="Invert RI 2", f=w384) -> (s? t:f=w387:bool)
              }
            }
            n150 = Subtract(x=w375, y=w347) -> (x-y=w358:u16)
            n151 = case shown="2" "Operating Mode 2" {
              tunnel: [TRUE FALSE w421] -> w334
              tunnel: w336 -> [_ _ w418]
              frame 0, Default {
              }
              frame 1 {
              }
              frame 2 {
                n152 = Not(x=w418) -> (.not. x?=w420:bool)
                n153 = Select(t=w420, s="Invert GI 2", f=w418) -> (s? t:f=w421:bool)
              }
            }
            n154 = Number To Boolean Array(number=w347) -> (Boolean array=w348:bool[])
            n155 = Boolean To (0,1)(Boolean="+ phase (GI) 2") -> (0, 1=w360:i16)
            n156 = Or Array Elements(Boolean array=w348) -> (logical OR=w346:bool)
            n157 = local read item#-1() -> (w331)
            n158 = Boolean To (0,1)(Boolean=w346) -> (0, 1=w353:i16)
            n159 = Multiply(x=w360, y="Phase count adjustment (GI) 2") -> (x*y=w356:i16)
            n160 = local read item#-1() -> (w333)
            n161 = local read "RF synth bd controls green"() -> (w328:bool)
            n162 = To Unsigned Byte Integer(number=w353) -> (unsigned 8bit integer=w349:u8)
            n163 = And(x=w331, y=w332) -> (x .and. y?=w330:bool)
            n164 = Add(x=w358, y=w356) -> (x+y=w354:u16)
            n165 = feedback #14(u8 0) -> (w351:u8)
            n166 = Add(x=w349, y=w351) -> (x+y=w350:u8)
            "GI Late Counter 2" <- w350
            n167 = feedback-in #14(w350) -> ()
            n168 = feedback #15(i16 0) -> (w357:i16)
            n169 = Subtract(x=w357, y=w356) -> (x-y=w355:i16)
            "GI Relative phase 2" <- w355
            n170 = feedback-in #15(w355) -> ()
            n171 = And(x=w334, y=w333) -> (x .and. y?=w335:bool)
            n172 = And(x=w335, y="Green FB On/Off") -> (x .and. y?=w365:bool)
            "green FB running" <- w365
            n173 = And(x=w330, y="Red FB On/Off") -> (x .and. y?=w345:bool)
            n174 = Not(x=w328) -> (.not. x?=w327:bool)
            n175 = case shown="True" w345 {
              tunnel: "RI Current Out" -> [w388 _]
              tunnel: [w388 w397] -> w341
              frame False {
              }
              frame True {
                n176 = local read "Red FB Intensity"() -> (w393:i16)
                n177 = Bundle("P4"="P4", "I4"="I4", "D4"="D4") -> (w389:cluster{"P4":i16, "I4":i16, "D4":i16})  [unwired: 1 in]
                n178 = call "Slower PID.vi"("process variable"=w393, "reset?"="Red FB Reset", "setpoint"="Red FB Setpoint", "PID gains (x 2^8)"=w389, "output range"=cluster{"output high":i16, "output low":i16} {"output high"=32767, "output low"=-32768} ("Green FB output range")) -> ("output"=w400:i16)  [unwired: 10 out]
                n179 = To Long Integer(number=w400) -> (32bit integer=w394:i32)
                n180 = Add(x=w394, y=32768) -> (x+y=w396:i32)
                n181 = To Unsigned Word Integer(number=w396) -> (unsigned 16bit integer=w397:u16)
              }
            }
            n182 = And(x=w365, y=w327) -> (x .and. y?=w329:bool)
            n183 = case shown="True" w329 {
              tunnel: "Current Out" -> [w402 w403]
              tunnel: [w402 w403] -> w369
              frame False {
              }
              frame True {
                n184 = disable-structure shown="Disabled" {
                  frame Disabled {
                    n185 = local read "Green FB Sum"() -> (w408:i16)
                    n186 = Bundle("P3"="P3", "I3"="I3", "D3"="D3") -> (w404:cluster{"P3":i16, "I3":i16, "D3":i16})  [unwired: 1 in]
                    n187 = call "Slower PID.vi"("process variable"=w408, "reset?"="Green FB Reset", "setpoint"="Green FB Setpoint", "PID gains (x 2^8)"=w404, "output range"=cluster{"output high":i16, "output low":i16} {"output high"=32767, "output low"=-32768} ("Green FB output range")) -> ("output"=w414:i16)  [unwired: 10 out]
                    n188 = To Long Integer(number=w414) -> (32bit integer=w409:i32)
                    n189 = Add(x=w409, y=32768) -> (x+y=w411:i32)
                    n190 = To Unsigned Word Integer(number=w411) -> ()  [unwired: 1 out]
                  }
                  frame Enabled {
                  }
                }
              }
            }
            n191 = Boolean To (0,1)(Boolean=w330) -> (0, 1=w340:i16)
            n192 = To Unsigned Word Integer(number=w340) -> (unsigned 16bit integer=w342:u16)
            n193 = Boolean To (0,1)(Boolean=w335) -> (0, 1=w371:i16)
            n194 = To Unsigned Word Integer(number=w371) -> (unsigned 16bit integer=w368:u16)
            n195 = Compound Arithmetic op=MULTIPLY(w342, w341) -> (w339:u16)
            n196 = Compound Arithmetic op=MULTIPLY(w368, w369) -> (w370:u16)
          }
        }
      }
      n197 = while "Blue fluorescent laser interlacing (AO control direct to laser)." {
        shift-right: [w241] -> _
        shift-left: w233 -> [w244]
        shift-right: [w238] -> _
        shift-left: i16 0 -> [w236]
        stop <- FALSE stop-if-true
        n198 = flat-sequence {
          tunnel: w244 -> [w247]
          tunnel: [w248] -> w243
          tunnel: [w247] -> w242
          tunnel: [w246] -> w237
          tunnel: w236 -> [w246]
          tunnel: [w251] -> w240
          tunnel: w243 -> [w251]
          tunnel: [w250] -> w239
          tunnel: w242 -> [w250]
          tunnel: w237 -> [w249]
          tunnel: [w261] -> w241
          tunnel: [w277] -> w238
          tunnel: w240 -> [w289]
          tunnel: w239 -> [w286]
          frame #0 {
            n199 = call "Loop Timer13"("Count(Ticks)"=w247) -> ("Tick Count(Ticks)"=w248:u16)
          }
          frame #1 {
            n200 = xnode "FPGA I/O Node"("Connector0/AO3"=w249) -> ()  [unwired: 1 in, 1 out]
          }
          frame #2 {
            n201 = Subtract(x="Blue OFF count (AO)", y="Blue current ON count adj (AO)") -> (x-y=w270:u16)
            n202 = feedback-in #16(w289) -> ()
            n203 = feedback #16(w289) -> (w288:u16)
            n204 = Add(x="Blue current ON count adj (AO)", y="Blue ON count (AO)") -> (x+y=w271:u16)
            n205 = Subtract(x=w289, y=w288) -> (x-y=w287:u16)
            n206 = Subtract(x=w287, y=w286) -> (x-y=w254:u16)
            n207 = Number To Boolean Array(number=w254) -> (Boolean array=w255:bool[])
            n208 = Boolean To (0,1)(Boolean="+ phase (BI AO)") -> (0, 1=w267:i16)
            n209 = Or Array Elements(Boolean array=w255) -> (logical OR=w253:bool)
            n210 = Boolean To (0,1)(Boolean=w253) -> (0, 1=w260:i16)
            n211 = Multiply(x=w267, y="Phase count adjustment (BI AO)") -> (x*y=w263:i16)
            n212 = To Unsigned Byte Integer(number=w260) -> (unsigned 8bit integer=w256:u8)
            n213 = feedback #17(u8 0) -> (w258:u8)
            n214 = Add(x=w256, y=w258) -> (x+y=w257:u8)
            "BI Late Counter (AO)" <- w257
            n215 = feedback-in #17(w257) -> ()
            n216 = feedback #18(i16 0) -> (w264:i16)
            n217 = Subtract(x=w264, y=w263) -> (x-y=w262:i16)
            "BI Relative phase (AO)" <- w262
            n218 = feedback-in #18(w262) -> ()
            n219 = feedback #19(TRUE) -> (w281:bool)
            n220 = case shown="2" "BI Operating Mode (AO)" {
              tunnel: [TRUE FALSE w305] -> w272
              tunnel: w281 -> [_ _ w302]
              frame 0, Default {
              }
              frame 1 {
              }
              frame 2 {
                n221 = Not(x=w302) -> (.not. x?=w304:bool)
                n222 = Select(t=w304, s="Invert BI (AO)", f=w302) -> (s? t:f=w305:bool)
              }
            }
            n223 = And(x=w272, y="Blue FB On/Off") -> (x .and. y?=w273:bool)
            n224 = case shown="True" w273 {
              tunnel: "BI Current Out" -> [w290 _]
              tunnel: [w290 w292] -> w276
              frame False {
              }
              frame True {
                n225 = local read "Blue Intensity"() -> (w291:i16)
                n226 = Bundle("P5"="P5", "I5"="I5", "D5"="D5") -> (w293:cluster{"P5":i16, "I5":i16, "D5":i16})  [unwired: 1 in]
                n227 = call "Slower PID.vi"("process variable"=w291, "reset?"="Blue FB Reset", "setpoint"="Blue FB Setpoint", "PID gains (x 2^8)"=w293, "output range"=cluster{"output high":i16, "output low":i16} {"output high"=32767, "output low"=0} ("Green FB output range")) -> ("output"=w292:i16)  [unwired: 10 out]
              }
            }
            n228 = Not(x=w281) -> (.not. x?=w278:bool)
            n229 = Select(t=w271, s=w278, f=w270) -> (s? t:f=w283:u16)
            n230 = Subtract(x=w283, y=w254) -> (x-y=w265:u16)
            n231 = Add(x=w265, y=w263) -> (x+y=w261:u16)
            n232 = feedback-in #19(w278) -> ()
            n233 = Boolean To (0,1)(Boolean=w272) -> (0, 1=w252:i16)
            n234 = Multiply(x=w252, y=w276) -> (x*y=w277:i16)
          }
        }
      }
    }
    frame Enabled {
    }
  }
  n235 = while "fluorescent laser interlacing (DO)." {
    shift-right: [w428] -> _
    shift-left: w2 -> [w433]
    shift-right: [w427] -> _
    shift-left: w14 -> [w425]
    shift-right: [w424] -> _
    shift-left: u8 0 -> [w422]
    stop <- FALSE stop-if-true
    n236 = flat-sequence {
      tunnel: w433 -> [w437]
      tunnel: [w438] -> w431
      tunnel: [w437] -> w429
      tunnel: [w436] -> w426
      tunnel: w425 -> [w436]
      tunnel: [w435] -> w423
      tunnel: w422 -> [w435]
      tunnel: [w442] -> w432
      tunnel: w431 -> [w442]
      tunnel: [w441] -> w430
      tunnel: w429 -> [w441]
      tunnel: w426 -> [w440]
      tunnel: w423 -> [w439]
      tunnel: [w471] -> w428
      tunnel: w432 -> [w490]
      tunnel: w430 -> [w487]
      tunnel: [w480] -> w427
      tunnel: [w452] -> w424
      frame #0 {
        n237 = call "Loop Timer4"("Count(Ticks)"=w437) -> ("Tick Count(Ticks)"=w438:u16)
      }
      frame #1 {
        n238 = case shown="2" w439 {
          tunnel: w440 -> [w444 w446 w448]
          frame 0, Default {
            w443 = FALSE
            n239 = xnode "FPGA I/O Node"("Connector0/DIO9"=w444, "Connector0/DIO11"=w443, "Connector0/DIO13"=w443) -> ()  [unwired: 3 in, 3 out]
          }
          frame 1 {
            w445 = FALSE
            n240 = xnode "FPGA I/O Node"("Connector0/DIO9"=w445, "Connector0/DIO11"=w446, "Connector0/DIO13"=w445) -> ()  [unwired: 3 in, 3 out]
          }
          frame 2 {
            w447 = FALSE
            n241 = xnode "FPGA I/O Node"("Connector0/DIO9"=w447, "Connector0/DIO11"=w447, "Connector0/DIO13"=w448) -> ()  [unwired: 3 in, 3 out]
          }
        }
      }
      frame #2 {
        # "Laser counting"
        n242 = feedback-in #20(w490) -> ()
        n243 = feedback #20(w490) -> (w489:u16)
        n244 = Subtract(x=w490, y=w489) -> (x-y=w488:u16)
        n245 = Subtract(x=w488, y=w487) -> (x-y=w464:u16)
        n246 = Number To Boolean Array(number=w464) -> (Boolean array=w465:bool[])
        n247 = Or Array Elements(Boolean array=w465) -> (logical OR=w463:bool)
        n248 = feedback #21(u8 0) -> (w461:u8)
        n249 = Increment(x=w461) -> (x+1=w458:u8)
        n250 = Less?(x=u8 5, y=w458) -> (x < y?=w459:bool)
        n251 = Select(t=u8 0, s=w459, f=w458) -> (s? t:f=w450:u8)
        n252 = feedback-in #21(w450) -> ()
        n253 = Boolean To (0,1)(Boolean=w463) -> (0, 1=w470:i16)
        n254 = Quotient & Remainder(x=w450, y=u8 2) -> (floor(x/y)=w449:u8)  [unwired: 1 out]
        n255 = To Unsigned Byte Integer(number=w470) -> (unsigned 8bit integer=w467:u8)
        n256 = feedback #22(u8 0) -> (w468:u8)
        n257 = Add(x=w467, y=w468) -> (x+y=w466:u8)
        "GI Late Counter" <- w466
        n258 = feedback-in #22(w466) -> ()
        n259 = Boolean To (0,1)(Boolean="+ phase (GI)") -> (0, 1=w476:i16)
        n260 = Multiply(x=w476, y="Phase count adjustment (GI)") -> (x*y=w473:i16)
        n261 = feedback #23(i16 0) -> (w474:i16)
        n262 = Subtract(x=w474, y=w473) -> (x-y=w472:i16)
        "GI Relative phase" <- w472
        n263 = feedback-in #23(w472) -> ()
        n264 = feedback #24(TRUE) -> (w483:bool)
        n265 = case shown="2" "Operating Mode" {
          tunnel: [TRUE FALSE w580] -> w480
          tunnel: w483 -> [_ _ w577]
          frame 0, Default {
          }
          frame 1 {
          }
          frame 2 {
            n266 = Not(x=w577) -> (.not. x?=w579:bool)
            n267 = Select(t=w579, s="Invert GI", f=w577) -> (s? t:f=w580:bool)
          }
        }
        n268 = Not(x=w483) -> (.not. x?=w479:bool)
        n269 = case shown="2" w449 {
          tunnel: "FL interlace ON count 0" -> [w500 w527 w554]
          tunnel: "FL interlace OFF count 0" -> [w499 w526 w553]
          tunnel: w479 -> [w498 w525 w556]
          tunnel: [w496 w524 w552] -> w477
          tunnel: w464 -> [w497 w528 w555]
          tunnel: "Fl interlace ON count 1" -> [w495 w523 w551]
          tunnel: "FL interlace OFF count 1" -> [w494 w522 w550]
          tunnel: "FL interlace ON count 2" -> [w493 w521 w549]
          tunnel: "FL interlace OFF count 2" -> [w492 w520 w548]
          tunnel: ["Laser choice 0" "Laser choice 1" "Laser choice 2"] -> w452
          frame 0, Default {
            n270 = case shown="1" "Laser choice 0" {
              tunnel: w500 -> [w505 _ _]
              tunnel: w499 -> [w504 _ _]
              tunnel: w498 -> [w503 w509 w515]
              tunnel: w497 -> [w502 w508 w514]
              tunnel: [w501 w507 w513] -> w496
              tunnel: w495 -> [_ w511 _]
              tunnel: w494 -> [_ w510 _]
              tunnel: w493 -> [_ _ w517]
              tunnel: w492 -> [_ _ w516]
              frame 0, Default {
                n271 = Select(t=w505, s=w503, f=w504) -> (s? t:f=w506:u16)
                n272 = Subtract(x=w506, y=w502) -> (x-y=w501:u16)
              }
              frame 1 {
                n273 = Select(t=w511, s=w509, f=w510) -> (s? t:f=w512:u16)
                n274 = Subtract(x=w512, y=w508) -> (x-y=w507:u16)
              }
              frame 2 {
                n275 = Select(t=w517, s=w515, f=w516) -> (s? t:f=w518:u16)
                n276 = Subtract(x=w518, y=w514) -> (x-y=w513:u16)
              }
            }
          }
          frame 1 {
            n277 = case shown="2" "Laser choice 1" {
              tunnel: w527 -> [w533 _ _]
              tunnel: w526 -> [w532 _ _]
              tunnel: w525 -> [w531 w537 w543]
              tunnel: w528 -> [w530 w536 w542]
              tunnel: [w529 w535 w541] -> w524
              tunnel: w523 -> [_ w539 _]
              tunnel: w522 -> [_ w538 _]
              tunnel: w521 -> [_ _ w545]
              tunnel: w520 -> [_ _ w544]
              frame 0, Default {
                n278 = Select(t=w533, s=w531, f=w532) -> (s? t:f=w534:u16)
                n279 = Subtract(x=w534, y=w530) -> (x-y=w529:u16)
              }
              frame 1 {
                n280 = Select(t=w539, s=w537, f=w538) -> (s? t:f=w540:u16)
                n281 = Subtract(x=w540, y=w536) -> (x-y=w535:u16)
              }
              frame 2 {
                n282 = Select(t=w545, s=w543, f=w544) -> (s? t:f=w546:u16)
                n283 = Subtract(x=w546, y=w542) -> (x-y=w541:u16)
              }
            }
          }
          frame 2 {
            n284 = case shown="2" "Laser choice 2" {
              tunnel: w554 -> [w561 _ _]
              tunnel: w553 -> [w560 _ _]
              tunnel: w556 -> [w559 w565 w571]
              tunnel: w555 -> [w558 w564 w570]
              tunnel: [w557 w563 w569] -> w552
              tunnel: w551 -> [_ w567 _]
              tunnel: w550 -> [_ w566 _]
              tunnel: w549 -> [_ _ w573]
              tunnel: w548 -> [_ _ w572]
              frame 0, Default {
                n285 = Select(t=w561, s=w559, f=w560) -> (s? t:f=w562:u16)
                n286 = Subtract(x=w562, y=w558) -> (x-y=w557:u16)
              }
              frame 1 {
                n287 = Select(t=w567, s=w565, f=w566) -> (s? t:f=w568:u16)
                n288 = Subtract(x=w568, y=w564) -> (x-y=w563:u16)
              }
              frame 2 {
                n289 = Select(t=w573, s=w571, f=w572) -> (s? t:f=w574:u16)
                n290 = Subtract(x=w574, y=w570) -> (x-y=w569:u16)
              }
            }
          }
        }
        n291 = Add(x=w477, y=w473) -> (x+y=w471:u16)
        n292 = feedback-in #24(w479) -> ()
      }
    }
  }
  n293 = while "DAQ AI set 1" {
    shift-right: [w581] -> _
    shift-left: w2 -> [w586]
    stop <- FALSE stop-if-true
    n294 = flat-sequence {
      tunnel: w586 -> [w596]
      tunnel: [w597] -> w584
      tunnel: [w596] -> w583
      tunnel: [w607] -> w594
      tunnel: [w606] -> w593
      tunnel: [w605] -> w592
      tunnel: [w604] -> w591
      tunnel: [w603] -> w590
      tunnel: [w602] -> w589
      tunnel: [w601] -> w588
      tunnel: [w600] -> w587
      tunnel: [w599] -> w585
      tunnel: w584 -> [w599]
      tunnel: w583 -> [w598]
      tunnel: [w598] -> w582
      tunnel: [w639] -> w581
      tunnel: w594 -> [w665]
      tunnel: w593 -> [w631]
      tunnel: w592 -> [w632]
      tunnel: w591 -> [w611]
      tunnel: w590 -> [w655]
      tunnel: w589 -> [w654]
      tunnel: w588 -> [w653]
      tunnel: w587 -> [w652]
      tunnel: w585 -> [w649]
      tunnel: w582 -> [w646]
      frame #0 {
        n295 = call "Loop Timer3"("Count(Ticks)"=w596) -> ("Tick Count(Ticks)"=w597:u16)
      }
      frame #1 {
        # "Signal changed to DIO15 to ease\nmeasurement in the room - change\nback for large code"
        n296 = xnode "FPGA I/O Node"("Connector0/DIO15"=TRUE ("Connector1/DIO33")) -> ("Connector0/AI0"=w607:i16, "Connector0/AI1"=w606:i16, "Connector0/AI2"=w605:i16, "Connector0/AI3"=w604:i16, "Connector0/AI4"=w603:i16, "Connector0/AI5"=w602:i16, "Connector0/AI6"=w601:i16, "Connector0/AI7"=w600:i16)  [unwired: 9 in, 9 out]
      }
      frame #2 {
        w635 = FALSE ("AI to FIFO")
        # "Normalize by trap bead QPD sum, AI3"
        # "Adjust phase after data acquired if button pressed"
        n297 = feedback #25(i16 1) -> (w658:i16)
        n298 = Increment(x=w658) -> (x+1=w664:i16)
        n299 = Scale By Power Of 2(n="AI1 X Scale", x=w631) -> (x*2^n=w629:i16)
        n300 = Greater?(x=w664, y="N of AI1 Int Acq Sets") -> (0:w661:bool)
        n301 = Select(t=i16 1, s=w661, f=w664) -> (s? t:f=w663:i16)
        n302 = feedback-in #25(w663) -> ()
        n303 = Divide(x=w629, y=w611) -> (x/y=w628:fxp<+/-,16,1>)
        n304 = feedback #26(w635) -> (w633:bool)
        n305 = feedback #27(w635) -> (w651:bool)
        n306 = case shown="1, Default" w658 {
          tunnel: w632 -> [w690 w697 _]
          tunnel: ["Set 1" "Set 2" "Set 3"] -> w656
          tunnel: ["AI to FIFO" w699 w704] -> w650
          tunnel: w651 -> [_ w699 w704]
          tunnel: ["Trap Pos to FIFO" w698 w703] -> w634
          tunnel: w633 -> [_ w698 w703]
          tunnel: w628 -> [w689 w696 _]
          tunnel: [w688 w694 FALSE] -> w615
          tunnel: [w687 w695 u64 0 ("BD1 Frequency Out 2")] -> w614
          frame 1, Default {
            n307 = local read "BD1 Frequency Out 1"() -> (w687:u64)
            n308 = Compound Arithmetic op=AND("Trap Pos to FIFO", "Set 1", "AI to FIFO") -> (w688:bool)
            "AI2 Y Sum Set 1" <- w690
            "AI1 X Set 1" <- w689
          }
          frame 2 {
            n309 = local read "BD1 Frequency Out 2"() -> (w695:u64)
            n310 = Compound Arithmetic op=AND(w698, "Set 2", w699) -> (w694:bool)
            "AI2 Y Sum Set 2" <- w697
            "AI1 X Set 2" <- w696
          }
          frame 3 {
          }
        }
        n311 = And(x=w656, y=w650) -> (x .and. y?=w657:bool)
        n312 = case shown="True" w657 {
          tunnel: w665 -> [_ w718]
          tunnel: w631 -> [_ w717]
          tunnel: w632 -> [_ w716]
          tunnel: w611 -> [_ w715]
          tunnel: w655 -> [_ w714]
          tunnel: w654 -> [_ w713]
          tunnel: w653 -> [_ w712]
          tunnel: w652 -> [_ w711]
          tunnel: 0 ("DMA buffer timeout") -> [_ w720]
          frame False {
          }
          frame True {
            n313 = Build Array(w718, w717, w716, w715, w714, w713, w712, w711) -> (w719:i16[])
            n314 = for {
              tunnel: w719 -> [w722] mode=indexing
              tunnel: w720 -> [w723]
              tunnel: [w721] -> w709 mode=indexing
              n315 = xnode ("FIFO Write")("Element"=w722, "Timeout"=w723) -> ("Timed Out?"=w721:bool)  [unwired: 1 in, 1 out]
            }
            n316 = Or Array Elements(Boolean array=w709) -> (logical OR=w706:bool)
            n317 = Boolean To (0,1)(Boolean=w706) -> (0, 1=w708:i16)
            n318 = feedback #28(u16 0) -> (w707:u16)
            n319 = Add(x=w708, y=w707) -> (x+y=w705:u16)
            "Trap AI FIFO Timeout" <- w705
            n320 = feedback-in #28(w705) -> ()
          }
        }
        n321 = feedback-in #26(w634) -> ()
        n322 = feedback-in #27(w650) -> ()
        n323 = local read "Piezo X out"() -> (w610:i16)
        n324 = local read "Piezo Y out"() -> (w609:i16)
        n325 = case shown="True" w615 {
          tunnel: w614 -> [_ w673]
          tunnel: [u8 0 w670] -> w613
          tunnel: w610 -> [_ w669]
          tunnel: w609 -> [_ w668]
          frame False {
          }
          frame True {
            n326 = Split Number(x=w673) -> (hi(x)=w674:u32, lo(x)=w675:u32)
            n327 = Split Number(x=w674) -> (lo(x)=w676:u16)  [unwired: 1 out]
            n328 = Split Number(x=w675) -> (hi(x)=w677:u16, lo(x)=w678:u16)
            n329 = Build Array "BD 1 nu Stack"(w676, w677, w678, w669, w668) -> (w672:u16[])
            n330 = for {
              tunnel: w672 -> [w685] mode=indexing
              shift-right: [w681] -> w670
              shift-left: u8 0 -> [w682]
              n331 = xnode ("FIFO Method Node")("Element"=w685, "Timeout"="Trap FIFO Set Timeout") -> ("Timed Out?"=w684:bool)  [unwired: 1 in, 1 out]
              n332 = Boolean To (0,1)(Boolean=w684) -> (0, 1=w683:i16)
              n333 = To Unsigned Byte Integer(number=w683) -> (unsigned 8bit integer=w680:u8)
              n334 = Add(x=w680, y=w682) -> (x+y=w681:u8)
            }
          }
        }
        n335 = To Unsigned Word Integer(number=w613) -> (unsigned 16bit integer=w612:u16)
        n336 = feedback #29(u16 0) -> (w626:u16)
        n337 = Add(x=w612, y=w626) -> (x+y=w625:u16)
        "Trap Pos FIFO Timeout" <- w625
        n338 = feedback-in #29(w625) -> ()
        n339 = feedback-in #30(w649) -> ()
        n340 = feedback #30(w649) -> (w648:u16)
        n341 = Subtract(x=w649, y=w648) -> (x-y=w647:u16)
        n342 = xnode "FPGA I/O Node"("Connector0/DIO15"=FALSE ("Connector1/DIO34")) -> ()  [unwired: 1 in, 1 out]
        n343 = Subtract(x=w647, y=w646) -> (x-y=w617:u16)
        n344 = Boolean To (0,1)(Boolean="+ phase") -> (0, 1=w642:i16)
        n345 = Multiply(x=w642, y="Phase count adjustment") -> (x*y=w636:i16)
        n346 = Subtract(x="ai count", y=w617) -> (x-y=w640:u16)
        n347 = Number To Boolean Array(number=w617) -> (Boolean array=w618:bool[])
        n348 = feedback #31(i16 0) -> (w638:i16)
        n349 = Add(x=w640, y=w636) -> (x+y=w639:u16)
        n350 = Subtract(x=w638, y=w636) -> (x-y=w637:i16)
        "Relative phase" <- w637
        n351 = feedback-in #31(w637) -> ()
        n352 = Or Array Elements(Boolean array=w618) -> (logical OR=w616:bool)
        n353 = Boolean To (0,1)(Boolean=w616) -> (0, 1=w623:i16)
        n354 = To Unsigned Byte Integer(number=w623) -> (unsigned 8bit integer=w620:u8)
        n355 = feedback #32(u8 0) -> (w621:u8)
        n356 = Add(x=w620, y=w621) -> (x+y=w619:u8)
        "AI Late Counter" <- w619
        n357 = feedback-in #32(w619) -> ()
      }
    }
  }
  n358 = while "MCL stage control" {
    shift-right: [w747] -> _
    shift-left: w2 -> [w750]
    shift-right: [w740] -> _
    shift-left: w12 -> [w737]
    shift-right: [w739] -> _
    shift-left: w11 -> [w735]
    shift-right: [w734] -> _
    shift-left: w10 -> [w729]
    shift-right: [w732] -> _
    shift-left: w10 -> [w724]
    shift-right: [w730] -> _
    shift-left: w10 -> [w726]
    stop <- FALSE stop-if-true
    n359 = flat-sequence {
      tunnel: w750 -> [w757]
      tunnel: [w758] -> w746
      tunnel: [w757] -> w744
      tunnel: [w756] -> w738
      tunnel: w737 -> [w756]
      tunnel: [w755] -> w736
      tunnel: w735 -> [w755]
      tunnel: w729 -> [w754]
      tunnel: [w754] -> w728
      tunnel: [w753] -> w727
      tunnel: w726 -> [w753]
      tunnel: [w752] -> w725
      tunnel: w724 -> [w752]
      tunnel: w746 -> [w765]
      tunnel: [w765] -> w745
      tunnel: w744 -> [w764]
      tunnel: [w764] -> w743
      tunnel: w738 -> [w763]
      tunnel: w736 -> [w762]
      tunnel: w728 -> [w761]
      tunnel: w727 -> [w760]
      tunnel: w725 -> [w759]
      tunnel: w745 -> [w779]
      tunnel: w743 -> [w778]
      tunnel: [w779] -> w749
      tunnel: [w778] -> w748
      tunnel: [w777] -> w742
      tunnel: [w776] -> w741
      tunnel: [w768] -> w733
      tunnel: [w766] -> w731
      tunnel: [w886] -> w747
      tunnel: w749 -> [w893]
      tunnel: w748 -> [w890]
      tunnel: w742 -> [w888]
      tunnel: w741 -> [w887]
      tunnel: [w888] -> w740
      tunnel: [w887] -> w739
      tunnel: [w869] -> w734
      tunnel: w733 -> [w869]
      tunnel: [w868] -> w732
      tunnel: w731 -> [w868]
      tunnel: ["Piezo Trap ON/Off (AO3)"] -> w730
      frame #0 {
        n360 = call "Loop Timer5"("Count(Ticks)"=w757) -> ("Tick Count(Ticks)"=w758:u32)
      }
      frame #1 {
        n361 = xnode "FPGA I/O Node"("Connector0/AO1"=w763, "Connector0/AO2"=w762, "Connector0/AO3"=w760, "Connector0/AO4"=w761, "Connector0/AO5"=w759) -> ()  [unwired: 5 in, 5 out]
      }
      frame #2 {
        n362 = local read "Scanning MCL"() -> (w791:bool)
        n363 = Or(x=w791, y="Start scan (MCL)") -> (x .or. y?=w786:bool)
        n364 = Not(x="Abort scan (MCL)") -> (.not. x?=w784:bool)
        n365 = And(x=w784, y=w786) -> (x .and. y?=w783:bool)
        n366 = case "Raster scan" shown="False" w783 {
          tunnel: [w824 w867] -> w788
          tunnel: "Start scan (MCL)" -> [_ w852]
          tunnel: [w824 w828] -> w772
          frame False {
            w824 = i16 0
            n367 = local write "Scanning MCL"(FALSE ("scanning")) -> ()
          }
          frame True {
            w838 = i16 0
            w837 = u64 0
            # "scan incr."
            # "freq. incr. mult."
            # "count steps"
            # "count number of cycles"
            n368 = feedback #33(w837) -> (w864:u64)
            n369 = Select(t=w837, s=w852, f=w864) -> (s? t:f=w866:u64)
            n370 = Increment(x=w866) -> (x+1=w863:u64)
            n371 = Greater?(x="Cycles per step (MCL)", y=w863) -> (0:w847:bool)
            n372 = Select(t=w863, s=w847, f=w837) -> (s? t:f=w862:u64)
            n373 = feedback-in #33(w862) -> ()
            n374 = feedback #34(w837) -> (w861:u64)
            n375 = Select(t=w837, s=w852, f=w861) -> (s? t:f=w856:u64)
            n376 = Increment(x=w856) -> (x+1=w860:u64)
            n377 = Add(x="Scan steps (MCL)", y="Scan steps (MCL)") -> (x+y=w859:u64)
            n378 = Select(t=w856, s=w847, f=w860) -> (s? t:f=w842:u64)
            n379 = Greater?(x=w859, y=w842) -> (0:w841:bool)
            n380 = Select(t=w842, s=w841, f=w837) -> (s? t:f=w857:u64)
            n381 = feedback-in #34(w857) -> ()
            n382 = Equal?(x="Scan steps (MCL)", y=w842) -> (x = y?=w846:bool)
            n383 = Greater?(x="Scan steps (MCL)", y=w856) -> (0:w855:bool)
            n384 = feedback #35(w838) -> (w858:i16)
            n385 = Select(t=w838, s=w852, f=w858) -> (s? t:f=w844:i16)
            n386 = Increment(x=w844) -> (x+1=w854:i16)
            n387 = Decrement(x=w844) -> (x-1=w853:i16)
            n388 = Select(t=w854, s=w855, f=w853) -> (s? t:f=w845:i16)
            n389 = Select(t=w844, s=w846, f=w845) -> (s? t:f=w843:i16)
            n390 = Select(t=w844, s=w847, f=w843) -> (s? t:f=w839:i16)
            n391 = Select(t=w839, s=w841, f=w838) -> (s? t:f=w840:i16)
            n392 = feedback-in #35(w840) -> ()
            n393 = feedback #36(w837) -> (w851:u64)
            n394 = Select(t=w837, s=w852, f=w851) -> (s? t:f=w826:u64)
            n395 = Increment(x=w826) -> (x+1=w848:u64)
            n396 = Select(t=w826, s=w841, f=w848) -> (s? t:f=w827:u64)
            n397 = Greater?(x="Number of scans (MCL)", y=w827) -> (0:w834:bool)
            n398 = Multiply(x="Scan freq.  increment (MCL)", y=w844) -> (x*y=w867:i16)
            n399 = Select(t=TRUE, s="Cont. Scan (MCL)", f=w834) -> (s? t:f=w833:bool)
            "Scanning MCL" <- w833
            n400 = Select(t=w827, s=w833, f=w837) -> (s? t:f=w849:u64)
            n401 = feedback-in #36(w849) -> ()
            n402 = Increment(x=w827) -> (x+1=→"Scan I (MCL)":u64)
            n403 = To Word Integer(number=w826) -> (16bit integer=w829:i16)
            n404 = Multiply(x=w829, y="Scan freq.  increment (MCL)") -> (x*y=w828:i16)
          }
        }
        n405 = case shown="True" "Multiple trap 3 position offset \nfile" {
          tunnel: ["Piezo Trap Y (AO4)" w811] -> w769
          tunnel: ["Piezo Trap X (AO5)" w810] -> w767
          frame False {
          }
          frame True {
            n406 = local read "Scan I"() -> (w822:u64)
            n407 = Decrement(x=w822) -> (x-1=w823:u64)
            n408 = Quotient & Remainder(x=w823, y="Piezo offset Y points") -> (x-y*floor(x/y)=w820:u64, floor(x/y)=w818:u64)
            n409 = Multiply(x=w820, y="Piezo Offset Increment") -> (x*y=w817:u64)
            n410 = Multiply(x="Piezo Offset Increment", y=w818) -> (x*y=w815:u64)
            n411 = Add(x=w815, y="Piezo offset Xmin") -> (x+y=w812:u64)
            n412 = Add(x=w817, y="Piezo Offset Ymin") -> (x+y=w813:u64)
            n413 = To Word Integer(number=w812) -> (16bit integer=w810:i16)
            n414 = To Word Integer(number=w813) -> (16bit integer=w811:i16)
          }
        }
        n415 = Select(t=w772, s="1D or 2D Scan?", f=i16 0) -> (s? t:f=w773:i16)
        n416 = Select(t=w788, s="MCL Scan Axis", f=w773) -> (s? t:f=w789:i16)
        n417 = Select(t=w773, s="MCL Scan Axis", f=w788) -> (s? t:f=w787:i16)
        n418 = case shown="True" "ScanTrap 3 or Fl-laser" {
          tunnel: w789 -> [w799 w801]
          tunnel: w787 -> [w794 w805]
          tunnel: "AO2 (X)" -> [w795 w806]
          tunnel: "AO1 (Y)" -> [w798 w807]
          tunnel: [w797 w807] -> w777
          tunnel: [w796 w806] -> w776
          tunnel: w769 -> [w793 w802]
          tunnel: [w793 w800] -> w768
          tunnel: w767 -> [w792 w804]
          tunnel: [w792 w803] -> w766
          frame False {
            n419 = Add(x=w795, y=w794) -> (x+y=w796:i16)
            n420 = Add(x=w798, y=w799) -> (x+y=w797:i16)
          }
          frame True {
            n421 = Add(x=w802, y=w801) -> (x+y=w800:i16)
            n422 = Add(x=w804, y=w805) -> (x+y=w803:i16)
          }
        }
      }
      frame #3 {
        n423 = feedback-in #37(w893) -> ()
        n424 = feedback #37(w893) -> (w892:u32)
        n425 = Boolean To (0,1)(Boolean="+ phase (MCL)") -> (0, 1=w884:i16)
        n426 = Subtract(x=w893, y=w892) -> (x-y=w891:u32)
        n427 = Multiply(x=w884, y="Phase count adjustment (MCL)") -> (x*y=w880:i16)
        n428 = Subtract(x=w891, y=w890) -> (x-y=w872:u32)
        n429 = Subtract(x="MCL count", y=w872) -> (x-y=w882:u32)
        n430 = feedback #38(i16 0) -> (w881:i16)
        n431 = Subtract(x=w881, y=w880) -> (x-y=w879:i16)
        "MCL Relative Phase" <- w879
        n432 = feedback-in #38(w879) -> ()
        n433 = Number To Boolean Array(number=w872) -> (Boolean array=w873:bool[])
        n434 = Or Array Elements(Boolean array=w873) -> (logical OR=w871:bool)
        n435 = Boolean To (0,1)(Boolean=w871) -> (0, 1=w878:i16)
        n436 = Add(x=w882, y=w880) -> (x+y=w886:u32)
        n437 = To Unsigned Byte Integer(number=w878) -> (unsigned 8bit integer=w875:u8)
        n438 = feedback #39(u8 0) -> (w876:u8)
        n439 = Add(x=w875, y=w876) -> (x+y=w874:u8)
        "MCL Late Counter" <- w874
        n440 = feedback-in #39(w874) -> ()
        "Piezo Y out" <- w869
        "Piezo X out" <- w868
      }
    }
  }
  n441 = while "Trap RF control, main calculations (raster scanning, intensity and position feedback, phase control etc) with primary timing trigger" {
    shift-right: [w909] -> _
    shift-left: w2 -> [w908]
    shift-right: [w907] -> _
    shift-left: FALSE ("Swap F1 and F2") -> [w906]
    shift-right: [w902] -> _
    shift-left: u16 0 ("BD 1 Amplitude 3") -> [w899]
    shift-right: [w901] -> _
    shift-left: u16 0 ("BD 2 Amplitude 3") -> [w897]
    shift-right: [w896] -> _
    shift-left: u64 0 -> [w895]
    stop <- FALSE stop-if-true
    n442 = flat-sequence {
      tunnel: w906 -> [w915]
      tunnel: w908 -> [w913]
      tunnel: [w915] -> w905
      tunnel: [w914] -> w904
      tunnel: [w913] -> w903
      tunnel: [w912] -> w900
      tunnel: w899 -> [w912]
      tunnel: [w911] -> w898
      tunnel: w897 -> [w911]
      tunnel: [w926] -> w909
      tunnel: [w925] -> w907
      tunnel: w905 -> [w924]
      tunnel: w904 -> [w923]
      tunnel: w903 -> [w922]
      tunnel: [w921] -> w902
      tunnel: [w920] -> w901
      tunnel: w900 -> [w919]
      tunnel: w898 -> [w918]
      tunnel: [w917] -> w896
      tunnel: w895 -> [w916]
      frame #0 {
        n443 = call "Loop Timer"("Count(Ticks)"=w913) -> ("Tick Count(Ticks)"=w914:u16)
      }
      frame #1 {
        n444 = flat-sequence {
          tunnel: w924 -> [w934]
          tunnel: w919 -> [w928]
          tunnel: w918 -> [w927]
          tunnel: [w996] -> w926
          tunnel: [w1008] -> w925
          tunnel: w923 -> [w1002]
          tunnel: w922 -> [w999]
          tunnel: [w945] -> w921
          tunnel: [w944] -> w920
          tunnel: [w936] -> w917
          tunnel: w916 -> [w935]
          frame #0 {
            w929 = -1 ("Timeout")
            # "Operation when you need a long delay for either X or Y to synchonize AOD light out phase (> ~100 ticks)\nor want shorter trap ON timing. Puts some of the delay timing in parallel with the later computations."
            # "Trigger the external loop by sending the boolean FSK value through a FIFO.\nTiming is precise."
            n445 = Boolean To (0,1)(Boolean=w934) -> (0, 1=w933:i16)
            n446 = To Unsigned Word Integer(number=w933) -> (unsigned 16bit integer=w932:u16)
            n447 = xnode ("FIFO Method Node")("Element"=w932, "Timeout"=w929) -> ("FIFO Out"=w931:refnum<k21>)  [unwired: 1 in, 1 out]
            n448 = xnode ("FIFO Method Node")("Element"=w928, "Timeout"=w929, "FIFO In"=w931) -> ("FIFO Out"=w930:refnum<k21>)  [unwired: 1 out]
            n449 = xnode ("FIFO Method Node")("Element"=w927, "Timeout"=w929, "FIFO In"=w930) -> ()  [unwired: 2 out]
          }
          frame #1 {
            # "Just counts, wraps around, 8 bit"
            # "Which trap cycle"
            # "Only save the 3rd set's amp in the loop"
            # "If this is NOT set 3 AND NOT (RF synth controls green AND green FB running)\nthen use this sets amp value (otherwise keep the green feedback value)"
            # "Just flips back and forth."
            # "If interlacing is off, this is which cycle to use."
            # "Keep track of trap cycles (trap 1, 2, 3...)"
            # "This is the prior cycle's on time"
            # "increment timing\nindex, reset to 0 if \nend of matrix"
            # "Reset to begginning (1) when number of cycles reached."
            # "timing index"
            # "build byte stacks for writing data\n(must correspond to addresses array constant)"
            # "Timing housekeeping"
            # "Adjust phase if late\n(maintains constant phase relationship between cycles)"
            n450 = feedback #40(u8 0 ("t")) -> (w1005:u8)
            n451 = Increment(x=w1005) -> (x+1=w1044:u8)
            n452 = Increment(x="Number Interlace Cycles") -> (x+1=w1039:u8)
            n453 = Equal?(x=w1044, y=w1039) -> (x = y?=w1046:bool)
            n454 = Select(t=u8 1, s=w1046, f=w1044) -> (s? t:f=w1004:u8)
            n455 = feedback-in #40(w1004) -> ()
            n456 = Increment(x=w1004) -> (x+1=w1041:u8)
            n457 = Equal?(x=w1041, y=w1039) -> (x = y?=w1042:bool)
            n458 = Select "This cycle"(t=u8 1, s=w1042, f=w1041) -> (s? t:f=w1038:u8)
            n459 = Select(t=w1038, s="Interlace ON/OFF", f="Interlace Off Parameters") -> (s? t:f=w955:u8)
            n460 = feedback-in #41(w1002) -> ()
            n461 = feedback #41(w1002) -> (w1001:u16)
            n462 = Select(t=w1004, s="Interlace ON/OFF", f="Interlace Off Parameters") -> (s? t:f=w1037:u8)
            n463 = Subtract(x=w1002, y=w1001) -> (x-y=w1000:u16)
            n464 = Subtract "The error"(x=w1000, y=w999) -> (x-y=w983:u16)
            n465 = case shown="1, Default" w1037 {
              tunnel: ["DIO count 1 (ticks)" "DIO count 2 (ticks)" "DIO count 3 (ticks)"] -> w998
              frame 1, Default {
              }
              frame 2 {
              }
              frame 3 {
              }
            }
            n466 = Number To Boolean Array(number=w983) -> (Boolean array=w984:bool[])
            n467 = Or Array Elements(Boolean array=w984) -> (logical OR=w982:bool)
            n468 = Boolean To (0,1)(Boolean=w982) -> (0, 1=w989:i16)
            n469 = To Unsigned Byte Integer(number=w989) -> (unsigned 8bit integer=w986:u8)
            n470 = feedback #42(u8 0) -> (w987:u8)
            n471 = Add(x=w986, y=w987) -> (x+y=w985:u8)
            "DIO Late Counter" <- w985
            n472 = feedback-in #42(w985) -> ()
            n473 = Subtract(x=w998, y=w983) -> (x-y=w997:u16)
            n474 = local read "green FB running"() -> (w968:bool)
            n475 = And(x=w968, y="RF synth bd controls green") -> (x .and. y?=w967:bool)
            n476 = feedback #43(i64 0 ("y")) -> (w980:i64)
            n477 = case "Synchronize trap oscillations - always begin/end with trap 1" shown="1, Default" w955 {
              tunnel: [w1152 w1153 w1154] -> w981
              tunnel: w980 -> [w1152 w1153 _]
              frame 2 {
              }
              frame 3 {
              }
              frame 1, Default {
                n478 = Or(x="Osc traps", y="Initiate trap osc") -> (x .or. y?=w1156:bool)
                n479 = case "Trap sine oscillation (or whatever pattern is stored in memory)" shown="True" w1156 {
                  tunnel: [i64 0 ("y") w1160] -> w1154
                  tunnel: "Initiate trap osc" -> [_ w1163]
                  frame False {
                  }
                  frame True {
                    w1167 = u16 0
                    w1165 = -1
                    n480 = local write "Initiate trap osc"(FALSE ("Initiate trap osc")) -> ()
                    n481 = feedback #44(w1167) -> (w1169:u16)
                    n482 = Select(t=w1167, s=w1163, f=w1169) -> (s? t:f=w1168:u16)
                    n483 = Greater Or Equal?(x=w1168, y="Trap osc period (pts)") -> (x >= y?=w1174:bool)
                    n484 = Or(x=w1163, y=w1174) -> (x .or. y?=w1175:bool)
                    n485 = Select(t=u16 0, s=w1175, f=w1168) -> (s? t:f=w1159:u16)
                    n486 = feedback #45(w1165) -> (w1166:i32)
                    n487 = Select(t=w1165, s=w1163, f=w1166) -> (s? t:f=w1164:i32)
                    n488 = Increment(x=w1164) -> (x+1=w1171:i32)
                    n489 = Equal?(x=w1159, y=u16 0) -> (x = y?=w1172:bool)
                    n490 = Increment(x=w1159) -> (x+1=w1179:u16)
                    n491 = feedback-in #44(w1179) -> ()
                    n492 = Select(t=w1171, s=w1172, f=w1164) -> (s? t:f=w1170:i32)
                    n493 = feedback-in #45(w1170) -> ()
                    n494 = case shown="False" "Osc trap cont." {
                      tunnel: w1170 -> [w1183 _]
                      frame False {
                        n495 = Greater Or Equal?(x=w1183, y="N trap osc periods") -> (x >= y?=w1181:bool)
                        n496 = Not(x=w1181) -> (.not. x?=w1180:bool)
                        n497 = local write "Osc traps"(w1180) -> ()
                      }
                      frame True {
                      }
                    }
                    n498 = xnode ("Memory Read")("Address"=w1159, "Memory In"=refnum<k21> "Trap osc memory") -> ("Data"=w1160:i64)  [unwired: 1 out]
                  }
                }
              }
            }
            n499 = case shown="1, Default" w955 {
              tunnel: [w1197 w1412 "BD 1 Frequency 3"] -> w1034
              tunnel: [w1247 w1411 w1437] -> w971
              tunnel: ["BD 2 Amplitude 1" "BD 2 Amplitude 2" w1436] -> w963
              tunnel: [w1194 w1408 "BD 1 Amplitude 3"] -> w945
              tunnel: "FB Gains" -> [w1217 w1418 _]
              tunnel: "FB output range" -> [w1218 w1417 _]
              tunnel: w981 -> [w1215 w1415 _]
              tunnel: "BD 2 Frequency 1" -> [w1212 _ _]
              tunnel: "BD 2 Frequency 2" -> [_ w1411 _]
              tunnel: "BD 2 Frequency 3" -> [_ _ w1437]
              tunnel: w967 -> [_ _ w1435]
              tunnel: [w1197 w1409 w1430] -> w936
              tunnel: w935 -> [w1196 w1409 w1430]
              frame 1, Default {
                w1232 = fxp<+/-,24,9> 0.0 ("AI1 X Set 2")
                w1226 = u16 0
                w1244 = u64 0 ("f")
                # "Changed by Ronen - correction \nby PID is now implemented not on \nthe Base BD1 frequency but on the last\nfrequency sent."
                # "Added by Ronen -\nUpper and Lower \nLimits for the FB \ngenerated frequency\nto avoid losing bead \nwhen tether breaks"
                # "Explanation of raster scanning:\n1. Cycles: increment counter by 1 every time interlace cycle returns to trap 1. As long as \n  Cycle per Step is larger than counter, keep incrementing counter and do not change step counter.\n  Once counter is equal to Cycles per step, zero counter and increment step counter.\n2. Steps: Increments up every time cycles counter equals cycles per step. Performs the following:\n- To determine DIRECTION of frequency change:  If ScanstepX2 is EQUAL to step counter (full for-back scan finished)\n   frequency increment is set to zero, AND step counter is set to zero. \n   Otherwise: if no change to step counter (because cycleperstep>cycle counter), then no change to frequency\n   increment. \n   If step counter has changed (cycleperstep=cycle counter), then need to figure out direction of frequency change:\n   if step counter is EQUAL to Scansteps: No change to frequency increment\n   Otherwise: If scan steps > step counter - 1 (forward scan NOT completed): increment frequency by 1\n                       If scan steps equal or smaller than step counter -1 (forward scan completed): increment frequency by -1\n\n3. Scans: Increment scan counter every time step counter equals 2Xscan steps (full for-back scan completed)\n    if number of scans > scan counter: Send TRUE to scanning, continue scan\n    if number of scans = scan counter: Send FALSE to Scanning, Scan finished.\n\n  The wire with the asterik can be used as the index for getting the mirror positions in the offset scan."
                # "This signal integration happens no matter what\nso that correct setpoints can be chosen before \nturning on the FB."
                # "Trap 1"
                n500 = local read "AI1 X Set 2"() -> (w1209:fxp<+/-,16,1>)
                n501 = local read "AI1 X Set 1"() -> (w1229:fxp<+/-,16,1>)
                n502 = local read "Scanning"() -> (w1248:bool)
                n503 = Multiply(x=w1209, y="B factor") -> (x*y=w1207:fxp<+/-,48,17>)
                n504 = Or(x=w1248, y="Start scan") -> (x .or. y?=w1242:bool)
                n505 = case shown="True" "Diff FB Measurement?" {
                  tunnel: w1207 -> [w1265 w1274]
                  tunnel: w1229 -> [w1264 w1275]
                  tunnel: [w1262 w1266] -> w1230
                  frame False {
                    n506 = Select(t=w1264, s="Trap Pos FB Monitor T1 or T2", f=w1265) -> (s? t:f=w1262:fxp<+/-,48,17>)
                  }
                  frame True {
                    n507 = Subtract(x=w1275, y=w1274) -> (x-y=w1267:fxp<+/-,48,17>)
                    n508 = Not(x="Negate Diff?") -> (.not. x?=w1273:bool)
                    n509 = Boolean To (0,1)(Boolean="Negate Diff?") -> (0, 1=w1271:i16)
                    n510 = Boolean To (0,1)(Boolean=w1273) -> (0, 1=w1272:i16)
                    n511 = Negate(x=w1271) -> (-x=w1270:i16)
                    n512 = Add(x=w1270, y=w1272) -> (x+y=w1268:i16)
                    n513 = Multiply(x=w1268, y=w1267) -> (x*y=w1266:fxp<+/-,63,32>)
                  }
                }
                n514 = Not(x="Abort scan") -> (.not. x?=w1240:bool)
                n515 = And(x=w1240, y=w1242) -> (x .and. y?=w1239:bool)
                n516 = case "For raster scanning" shown="True" w1239 {
                  tunnel: [u64 0 w1398] -> w1245
                  tunnel: "Start scan" -> [_ w1383]
                  tunnel: [u64 1 w1360] -> w1210
                  frame False {
                    n517 = local write "Scanning"(FALSE ("scanning")) -> ()
                  }
                  frame True {
                    w1367 = i64 0
                    w1366 = u64 0
                    # "scan incr."
                    # "freq. incr. mult."
                    # "count steps"
                    # "count number of cycles"
                    n518 = feedback #46(w1366) -> (w1395:u64)
                    n519 = Select(t=w1366, s=w1383, f=w1395) -> (s? t:f=w1397:u64)
                    n520 = Increment(x=w1397) -> (x+1=w1394:u64)
                    n521 = Greater?(x="Cycles per step", y=w1394) -> (0:w1376:bool)
                    n522 = Select(t=w1394, s=w1376, f=w1366) -> (s? t:f=w1393:u64)
                    n523 = feedback-in #46(w1393) -> ()
                    n524 = feedback #47(w1366) -> (w1392:u64)
                    n525 = Select(t=w1366, s=w1383, f=w1392) -> (s? t:f=w1387:u64)
                    n526 = Increment(x=w1387) -> (x+1=w1391:u64)
                    n527 = Add(x="Scan steps", y="Scan steps") -> (x+y=w1390:u64)
                    n528 = Select(t=w1387, s=w1376, f=w1391) -> (s? t:f=w1371:u64)
                    n529 = Greater?(x=w1390, y=w1371) -> (0:w1370:bool)
                    n530 = Select(t=w1371, s=w1370, f=w1366) -> (s? t:f=w1388:u64)
                    n531 = feedback-in #47(w1388) -> ()
                    n532 = Equal?(x="Scan steps", y=w1371) -> (x = y?=w1375:bool)
                    n533 = Greater?(x="Scan steps", y=w1387) -> (0:w1386:bool)
                    n534 = feedback #48(w1367) -> (w1389:i64)
                    n535 = Select(t=w1367, s=w1383, f=w1389) -> (s? t:f=w1373:i64)
                    n536 = Increment(x=w1373) -> (x+1=w1385:i64)
                    n537 = Decrement(x=w1373) -> (x-1=w1384:i64)
                    n538 = Select(t=w1385, s=w1386, f=w1384) -> (s? t:f=w1374:i64)
                    n539 = Select(t=w1373, s=w1375, f=w1374) -> (s? t:f=w1372:i64)
                    n540 = Select(t=w1373, s=w1376, f=w1372) -> (s? t:f=w1368:i64)
                    n541 = Select(t=w1368, s=w1370, f=w1367) -> (s? t:f=w1369:i64)
                    n542 = feedback-in #48(w1369) -> ()
                    n543 = feedback #49(w1366) -> (w1382:u64)
                    n544 = Select(t=w1366, s=w1383, f=w1382) -> (s? t:f=w1378:u64)
                    n545 = Increment(x=w1378) -> (x+1=w1379:u64)
                    n546 = Select(t=w1378, s=w1370, f=w1379) -> (s? t:f=w1377:u64)
                    n547 = Greater?(x="Number of scans", y=w1377) -> (0:w1363:bool)
                    n548 = Multiply(x="Scan freq.  increment", y=w1373) -> (x*y=w1398:i64)
                    n549 = Select(t=TRUE, s="Cont. Scan", f=w1363) -> (s? t:f=w1362:bool)
                    "Scanning" <- w1362
                    n550 = Select(t=w1377, s=w1362, f=w1366) -> (s? t:f=w1380:u64)
                    n551 = feedback-in #49(w1380) -> ()
                    n552 = Increment(x=w1377) -> (x+1=w1360:u64)
                  }
                }
                "Scan I" <- w1210
                n553 = feedback #50(w1226) -> (w1225:u16)
                n554 = Increment(x=w1225) -> (x+1=w1227:u16)
                n555 = Greater Or Equal?(x=w1227, y="Trap Pos FB Int Count") -> (x >= y?=w1195:bool)
                n556 = Select(t=w1226, s=w1195, f=w1227) -> (s? t:f=w1228:u16)
                n557 = feedback-in #50(w1228) -> ()
                n558 = feedback #51(w1232) -> (w1231:fxp<+/-,24,9>)
                n559 = Add(x=w1230, y=w1231) -> (x+y=w1224:fxp<+/-,24,9>)
                n560 = case "Trap 1 X intensity feedback" shown="True" "FB On/Off Set 1" {
                  tunnel: "BD 1 Amplitude 1" -> [w1400 _]
                  tunnel: [w1400 w1404] -> w1194
                  tunnel: w1218 -> [_ w1401]
                  tunnel: w1217 -> [_ w1402]
                  frame False {
                  }
                  frame True {
                    n561 = local read "AI2 Y Sum Set 1"() -> (w1405:i16)
                    n562 = call "Slower PID.vi"("process variable"=w1405, "reset?"="FB Reset Set 1", "setpoint"="FB Setpoint Set 1", "PID gains (x 2^8)"=w1402, "output range"=w1401) -> ("output"=w1406:i16)  [unwired: 10 out]
                    n563 = To Unsigned Word Integer(number=w1406) -> (unsigned 16bit integer=w1404:u16)
                  }
                }
                "BD1 amplitude 1 out" <- w1194
                n564 = Select(t=w1232, s=w1195, f=w1224) -> (s? t:f=w1235:fxp<+/-,24,9>)
                n565 = feedback-in #51(w1235) -> ()
                n566 = Divide(x=w1224, y="Trap Pos FB Int Count") -> (x/y=w1219:fxp<+/-,16,1>)
                n567 = feedback #52(fxp<+/-,24,9> 0.0 ("AI1 X Set 2")) -> (w1236:fxp<+/-,24,9>)
                n568 = Select(t=w1224, s=w1195, f=w1236) -> (s? t:f=w1237:fxp<+/-,24,9>)
                "Trap Pos FB Int Signal" <- w1237
                n569 = feedback-in #52(w1237) -> ()
                n570 = feedback #53(fxp<+/-,16,1> 0.0 ("Trap Pos FB Int-Norm Signal")) -> (w1221:fxp<+/-,16,1>)
                n571 = Select(t=w1219, s=w1195, f=w1221) -> (s? t:f=w1220:fxp<+/-,16,1>)
                "Trap Pos FB Int-Norm Signal" <- w1220
                n572 = feedback-in #53(w1220) -> ()
                n573 = case "For position feedback" shown="True" "Force feedback" {
                  tunnel: [i64 0 w1281] -> w1202
                  tunnel: w1219 -> [_ w1278]
                  tunnel: w1195 -> [_ w1277]
                  frame False {
                  }
                  frame True {
                    n574 = feedback #54(i64 0) -> (w1280:i64)
                    n575 = case shown="False" w1277 {
                      tunnel: [w1282 w1286] -> w1281
                      tunnel: w1280 -> [w1282 _]
                      tunnel: w1278 -> [_ w1285]
                      frame False {
                      }
                      frame True {
                        n576 = xnode ("PID")("process variable"=w1285, "reset?"="Trap Pos. FB Reset", "setpoint"="Trap Pos. FB SP", "PID gains"="Trap Pos. FB Gains", "output range"="Trap pos. FB Range") -> ("output"=w1295:fxp<+/-,16,1>)
                        n577 = Negate(x=w1295) -> (-x=w1294:fxp<+/-,17,2>)
                        n578 = Select(t=w1294, s="Trap Pos FB Negate Action", f=w1295) -> (s? t:f=w1291:fxp<+/-,17,2>)
                        n579 = Scale By Power Of 2(n=u32 15, x=u32 1) -> (x*2^n=w1288:u32)
                        n580 = Multiply(x=w1291, y=w1288) -> (x*y=w1287:fxp<+/-,17,17>)
                        n581 = To Quad Integer(1:w1287) -> (0:w1299:i64)
                        "Trap Pos FB Action" <- w1299
                        n582 = Multiply(x=w1299, y="Trap Pos. FB Mult Factor") -> (x*y=w1297:i64)
                        n583 = Add(x=w1297, y="Trap Pos. FB Offset Factor") -> (x+y=w1286:i64)
                        n584 = disable-structure shown="Disabled" {
                          disable-tunnel: w1286 -> [w1306 _]
                          frame Disabled {
                            w1310 = u32 0
                            n585 = feedback #55() -> (w1307:i64)  [unwired: 1 in]
                            n586 = Add(x=w1306, y=w1307) -> (x+y=w1304:i64)
                            n587 = feedback #56(w1310) -> (w1312:u32)
                            n588 = Increment(x=w1312) -> (x+1=w1301:u32)
                            n589 = Greater Or Equal?(x=w1301, y="FB Trig Integrate") -> (x >= y?=w1302:bool)
                            n590 = Select(t=i64 0, s=w1302, f=w1304) -> (s? t:f=w1308:i64)
                            n591 = feedback-in #55(w1308) -> ()
                            n592 = Select(t=w1310, s=w1302, f=w1301) -> (s? t:f=w1311:u32)
                            n593 = feedback-in #56(w1311) -> ()
                            n594 = And(x=w1302, y="FPGA Trap Trig") -> (x .and. y?=w1309:bool)
                            n595 = case "Trap FB trigger excitation laser ON" shown="True" w1309 {
                              tunnel: w1304 -> [_ w1316]
                              tunnel: w1301 -> [_ w1314]
                              frame False {
                              }
                              frame True {
                                n596 = Not(x="TTrig Negate Pos") -> (.not. x?=w1323:bool)
                                n597 = Boolean To (0,1)(Boolean="TTrig Negate Pos") -> (0, 1=w1321:i16)
                                n598 = Boolean To (0,1)(Boolean=w1323) -> (0, 1=w1322:i16)
                                n599 = Negate(x=w1321) -> (-x=w1320:i16)
                                n600 = Add(x=w1320, y=w1322) -> (x+y=w1319:i16)
                                n601 = Multiply(x=w1319, y=w1316) -> (x*y=w1318:i64)
                                "TTrig Sig" <- w1318
                                n602 = Multiply(x="FPGA TTrig Thresh", y=w1314) -> (x*y=w1315:i64)
                                "TTrig Fin Thresh" <- w1315
                                n603 = Greater Or Equal?(x=w1318, y=w1315) -> (x >= y?=w1317:bool)
                                n604 = case shown="True" w1317 {
                                frame False {
                                }
                                frame True {
                                w1326 = TRUE ("Green FB On/Off")
                                w1328 = u8 2 ("Operating Mode")
                                n605 = local write "Operating Mode 2"(w1328) -> ()
                                n606 = local write "Operating Mode"(w1328) -> ()
                                n607 = local write "Green FB On/Off"(w1326) -> ()
                                n608 = local write "FPGA Trap Trig"(FALSE ("FPGA Trap Trig")) -> ()
                                "TTrig?" <- w1326
                                }
                                }
                              }
                            }
                          }
                          frame Enabled {
                          }
                        }
                      }
                    }
                    n609 = feedback-in #54(w1281) -> ()
                  }
                }
                n610 = And(x="Force feedback", y="Dynamic Force FB (Ronen)") -> (x .and. y?=w1204:bool)
                n611 = case shown="True" w1204 {
                  tunnel: w1202 -> [w1253 w1257]
                  tunnel: [w1252 w1256] -> w1203
                  tunnel: w1196 -> [_ w1255]
                  tunnel: w1195 -> [_ w1254]
                  frame False {
                    # "(BD1 Frequency 1)"
                    n612 = Add(x="BD 1 Frequency 1", y=w1253) -> (x+y=w1252:u64)
                  }
                  frame True {
                    n613 = case shown="True" w1254 {
                      tunnel: w1257 -> [_ w1261]
                      tunnel: [w1258 w1260] -> w1256
                      tunnel: w1255 -> [w1258 w1259]
                      frame False {
                      }
                      frame True {
                        n614 = Add(x=w1259, y=w1261) -> (x+y=w1260:u64)
                      }
                    }
                  }
                }
                n615 = Select(t=w1215, s="Trap 1 osc enable", f=i64 0) -> (s? t:f=w1213:i64)
                n616 = Select(t=w1244, s="Scan BD", f=w1245) -> (s? t:f=w1243:u64)
                n617 = Select(t=w1245, s="Scan BD", f=w1244) -> (s? t:f=w1201:u64)
                n618 = Add(x=w1243, y=w1212) -> (x+y=w1247:u64)
                n619 = Compound Arithmetic op=ADD(w1213, w1203, w1201) -> (w1200:u64)
                n620 = In Range and Coerce(upper limit="FB Max Frequency", x=w1200, lower limit="FB Min frequency") -> (coerced(x)=w1197:u64)  [unwired: 1 out]
                "BD1 Frequency Out 1" <- w1197
              }
              frame 2 {
                # "Trap 2"
                n621 = case "Trap 2 X intensity feedback" shown="True" "FB On/Off Set 2" {
                  tunnel: [w1422 w1425] -> w1408
                  tunnel: "BD 1 Amplitude 2" -> [w1422 _]
                  tunnel: w1418 -> [_ w1424]
                  tunnel: w1417 -> [_ w1423]
                  frame False {
                  }
                  frame True {
                    n622 = local read "AI2 Y Sum Set 2"() -> (w1428:i16)
                    n623 = call "Slower PID.vi"("process variable"=w1428, "reset?"="FB Reset Set 2", "setpoint"="FB Setpoint Set 2", "PID gains (x 2^8)"=w1424, "output range"=w1423) -> ("output"=w1426:i16)  [unwired: 10 out]
                    n624 = To Unsigned Word Integer(number=w1426) -> (unsigned 16bit integer=w1425:u16)
                  }
                }
                "BD1 amplitude 2 out" <- w1408
                n625 = Select(t=w1415, s="Trap 2 osc enable", f=i64 0) -> (s? t:f=w1414:i64)
                n626 = Add(x="BD 1 Frequency 2", y=w1414) -> (x+y=w1412:u64)
                "BD1 Frequency Out 2" <- w1412
              }
              frame 3 {
                # "Remember if FB was previously on/off"
                # "Fluorescence period"
                n627 = feedback #57(FALSE) -> (w1431:bool)
                n628 = case shown="True" w1435 {
                  tunnel: [w1441 w1457] -> w1436
                  tunnel: "BD 2 Amplitude 3" -> [w1441 _]
                  tunnel: [FALSE TRUE] -> w1432
                  tunnel: w1431 -> [_ w1442]
                  frame False {
                  }
                  frame True {
                    # "Makes it so first time FB run when turned on, the PID sees the detector intensity from the last time FB was running, rather than something near zero. Especially assuming the setpoint is not changing, this will make the FB more stable when resuming, and not overshoot the turnon intensity."
                    # "FB output range: 0 should be low, full scale is 12 bits.\nBut be careful not to go over, then higher bits just get ignored by RF board, so output will actually jump down and be unstable. Keep it under 4000 to be safe."
                    n629 = local read "Green FB Sum"() -> (w1445:i16)
                    n630 = feedback-in #58(w1445) -> ()
                    n631 = feedback #58(i16 0 ("Green FB Sum")) -> (w1444:i16)
                    n632 = Select(t=w1445, s=w1442, f=w1444) -> (s? t:f=w1443:i16)
                    n633 = Bundle("P3 2"="P3 2", "I3 2"="I3 2", "D3 2"="D3 2") -> (w1456:cluster{"P3 2":i16, "I3 2":i16, "D3 2":i16})  [unwired: 1 in]
                    n634 = Bundle("RF synth green feedback max"="RF synth green feedback max", i16 0) -> (w1448:cluster{"RF synth green feedback max":i16, i16})  [unwired: 1 in]
                    n635 = call "Slower PID.vi"("process variable"=w1443, "reset?"="Green FB Reset 2", "setpoint"="Green FB Setpoint 2", "PID gains (x 2^8)"=w1456, "output range"=w1448) -> ("output"=w1458:i16)  [unwired: 10 out]
                    n636 = To Unsigned Word Integer(number=w1458) -> (unsigned 16bit integer=w1457:u16)
                  }
                }
                n637 = feedback-in #57(w1432) -> ()
              }
            }
            n638 = feedback-in #43(w981) -> ()
            n639 = Split Number(x=w1034) -> (hi(x)=w1033:u32, lo(x)=w1032:u32)
            n640 = Boolean To (0,1)(Boolean="+ phase (DIO)") -> (0, 1=w994:i16)
            n641 = Split Number(x=w1033) -> (lo(x)=w1031:u16)  [unwired: 1 out]
            n642 = Split Number(x=w1032) -> (hi(x)=w1030:u16, lo(x)=w1029:u16)
            n643 = Split Number(x=w1031) -> (hi(x)=w1023:u8, lo(x)=w1022:u8)
            n644 = Split Number(x=w1030) -> (hi(x)=w1021:u8, lo(x)=w1020:u8)
            n645 = Split Number(x=w1029) -> (hi(x)=w1019:u8, lo(x)=w1018:u8)
            n646 = Multiply(x=w994, y="Phase count adjustment (DIO)") -> (x*y=w990:i16)
            n647 = feedback #59(TRUE) -> (w977:bool)
            n648 = Not(x=w977) -> (.not. x?=w976:bool)
            n649 = feedback-in #59(w976) -> ()
            n650 = feedback #60(i16 0) -> (w992:i16)
            n651 = Subtract(x=w992, y=w990) -> (x-y=w991:i16)
            "DIO Relative phase" <- w991
            n652 = feedback-in #60(w991) -> ()
            n653 = Add(x=w997, y=w990) -> (x+y=w996:u16)
            n654 = Build Array "BD 1 nu Stack"(w1023, w1022, w1021, w1020, w1019, w1018) -> (w1017:u8[])
            n655 = Not Equal?(x=w955, y=u8 3) -> (x != y?=w964:bool)
            n656 = case "Store in RF board F1 or F2" shown="True" w976 {
              tunnel: [w1185 w1189] -> w1008
              tunnel: [u8 10 u8 4] -> w1009
              tunnel: "Swap F1 and F2" -> [w1186 w1189]
              tunnel: "BD 2 Frequency 1" -> [_ w1188]
              tunnel: "BD 2 Frequency 2" -> [w1184 _]
              tunnel: [w1184 w1188] -> w972
              frame False {
                # "for RF synth controls\ngreen: F1/F2 stay same"
                # "F2 address (hex)"
                n657 = Not(x=w1186) -> (.not. x?=w1185:bool)
              }
              frame True {
                # "low chooses F1"
                # "F1 address (hex)"
              }
            }
            n658 = Select(t=w972, s="RF synth bd controls green", f=w971) -> (s? t:f=w970:u64)
            n659 = Split Number(x=w970) -> (hi(x)=w1028:u32, lo(x)=w1027:u32)
            n660 = Split Number(x=w1028) -> (lo(x)=w1026:u16)  [unwired: 1 out]
            n661 = Split Number(x=w1027) -> (hi(x)=w1025:u16, lo(x)=w1024:u16)
            n662 = Split Number(x=w1026) -> (hi(x)=w1016:u8, lo(x)=w1015:u8)
            n663 = Split Number(x=w1025) -> (hi(x)=w1014:u8, lo(x)=w1013:u8)
            n664 = Split Number(x=w1024) -> (hi(x)=w1012:u8, lo(x)=w1011:u8)
            n665 = feedback #61(u16 0 ("BD 2 Amplitude 3")) -> (w961:u16)
            n666 = Select(t=w961, s=w964, f=w963) -> (s? t:f=w962:u16)
            n667 = feedback-in #61(w962) -> ()
            n668 = And(x=w964, y=w967) -> (x .and. y?=w966:bool)
            n669 = Build Array "BD 2 nu Stack"(w1016, w1015, w1014, w1013, w1012, w1011) -> (w1010:u8[])
            n670 = Select(t=w961, s=w966, f=w963) -> (s? t:f=w944:u16)
            n671 = flat-sequence "Update trap RF synth board settings to be used for the upcoming trap cycle." {
              tunnel: w1010 -> [w1101]
              tunnel: w1017 -> [w1102]
              tunnel: [w1102] -> w959
              tunnel: [w1101] -> w958
              tunnel: w1009 -> [w1103]
              tunnel: w959 -> [w1105]
              tunnel: w958 -> [w1104]
              tunnel: w946 -> [w1116]
              tunnel: w948 -> [w1115]
              tunnel: w947 -> [w1114]
              frame #0 {
                # "To possibly delay\nthese writes to very\nend of loop (for x and\ny phase adjust)"
                n672 = call "Wait8"("Count(Ticks)"="Next trap write delay (ticks)") -> ()  [unwired: 1 out]
              }
              frame #1 {
                # "Next trap RF frequency:\n\nWrite next trap cycle frequency to buffer."
                n673 = for {
                  tunnel: w1105 -> [w1111] mode=indexing
                  tunnel: w1104 -> [w1110] mode=indexing
                  tunnel: w1103 -> [w1108]
                  i -> [w1109]
                  n674 = To Unsigned Byte Integer(number=w1109) -> (unsigned 8bit integer=w1106:u8)
                  n675 = Add(x=w1108, y=w1106) -> (x+y=w1107:u8)
                  n676 = call "write to RF synth bd.vi"("Address Byte"=w1107, "BD 2 Byte"=w1110, "BD 1 Byte"=w1111) -> ()
                }
              }
              frame #2 {
                w1112 = TRUE ("Connector1/DIO15")
                # "Send udclk high\n(BD 1 and 2) to make the new frequency active in F1 or F2 word. But it won't actually be the used frequency until FSK switches to it (begining of next cycle)."
                n677 = xnode "FPGA I/O Node"("Connector1/DIO30"=w1112, "Connector1/DIO29"=w1112) -> ()  [unwired: 2 in, 2 out]
              }
              frame #3 {
                w1113 = FALSE ("Connector1/DIO15")
                n678 = xnode "FPGA I/O Node"("Connector1/DIO30"=w1113, "Connector1/DIO29"=w1113) -> ()  [unwired: 2 in, 2 out]
              }
              frame #4 {
                # "Next trap RF phase offset:\n\nSet the next trap cycle amplitude to the buffer. Won't become active until udclk is set high at proper time at the begining of the next cycle."
                n679 = case shown="True" w1116 {
                  tunnel: w1115 -> [_ w1117]
                  tunnel: w1114 -> [_ w1118]
                  frame False {
                  }
                  frame True {
                    # "phase 1 address start"
                    n680 = for {
                      tunnel: w1117 -> [w1125] mode=indexing
                      tunnel: w1118 -> [w1124] mode=indexing
                      tunnel: u8 0 -> [w1122]
                      i -> [w1123]
                      n681 = To Unsigned Byte Integer(number=w1123) -> (unsigned 8bit integer=w1120:u8)
                      n682 = Add(x=w1122, y=w1120) -> (x+y=w1121:u8)
                      n683 = call "write to RF synth bd.vi"("Address Byte"=w1121, "BD 2 Byte"=w1124, "BD 1 Byte"=w1125) -> ()
                    }
                  }
                }
              }
              frame #5 {
                # "Prep to reset RF phase to zero at start of next cycle. Only reset BD 1. Do nothing to BD 2. This puts the settings in the buffer. A udclk high will make both this phase reset and possibly a new phase offset setting active."
                n684 = case shown="True" "RF phase reset before cycles" {
                  frame False {
                  }
                  frame True {
                    w1128 = u8 66  # BD 1 reset
                    n685 = call "write to RF synth bd.vi"("Address Byte"=u8 31, "BD 2 Byte"=u8 2, "BD 1 Byte"=w1128) -> ()
                  }
                }
              }
              frame #6 {
                # "Address"
                # "Data BD 2"
                # "Data BD 1"
                # "If phase reset wasn't chosen previously, these actions will have no affect. For both BD's, data should be binary 10, and address should be hex 1F (bin 01 1111)"
                # "This sets up the digital communication lines to restart phase accumulation (start RF running agin). It cancels out the possible phase reset. Just need to set WR DIO low then udclk DIOhigh  to make this happen. Doing this here early (and not using the usual board write function) speeds things up.\n\nRestarts RF (BD 1 only, BD2 never stopped in first place)."
                n686 = xnode "FPGA I/O Node"("Connector1/DIO0"=FALSE, "Connector1/DIO1"=FALSE, "Connector1/DIO2"=FALSE, "Connector1/DIO3"=FALSE, "Connector1/DIO4"=FALSE, "Connector1/DIO5"=FALSE, "Connector1/DIO6"=TRUE, "Connector1/DIO7"=FALSE, "Connector1/DIO8"=FALSE, "Connector1/DIO9"=TRUE, "Connector1/DIO10"=TRUE, "Connector1/DIO11"=TRUE, "Connector1/DIO12"=TRUE, "Connector1/DIO13"=TRUE, "Connector1/DIO20"=FALSE, "Connector1/DIO21"=FALSE, "Connector1/DIO22"=FALSE, "Connector1/DIO23"=FALSE, "Connector1/DIO24"=FALSE, "Connector1/DIO25"=FALSE, "Connector1/DIO26"=TRUE, "Connector1/DIO27"=FALSE) -> ()  [unwired: 22 in, 22 out]
              }
            }
            n687 = feedback #62(fxp<+,8,8> 0.0) -> (w941:fxp<+,8,8>)
            n688 = Increment(x=w941) -> (x+1=w939:fxp<+,8,8>)
            n689 = feedback-in #62(w939) -> ()
            n690 = case "Trap RF phase offset control methods" shown="3" "Phase offset method" {
              tunnel: [fxp<+,14,14> 0.0 ("Phase BD 1") w1051 w1066 w1095] -> w949
              tunnel: "Phase Trap 1" -> [_ w1052 w1067 _]
              tunnel: w955 -> [_ w1053 w1068 w1096]
              tunnel: [FALSE TRUE TRUE TRUE] -> w946
              tunnel: "Phase Trap 2" -> [_ w1049 w1064 _]
              tunnel: w939 -> [_ _ w1063 _]
              frame 0, Default {
              }
              frame 1 {
                # "Constant increment of phase offset with each trap cycle. This results in a constant phase difference between trap cycles. \nOnly for traps 1 and 2 (set phase offset to zero for set three)."
                n691 = case shown="1, Default" w1053 {
                  tunnel: w1052 -> [_ _ w1059]
                  tunnel: [w1055 fxp<+,14,14> 0.0 w1060] -> w1051
                  tunnel: w1049 -> [w1054 _ _]
                  frame 2 {
                    n692 = feedback #63(fxp<+,14,14> 0.0) -> (w1057:fxp<+,14,14>)
                    n693 = Add(x=w1054, y=w1057) -> (x+y=w1055:fxp<+,14,14>)
                    n694 = feedback-in #63(w1055) -> ()
                  }
                  frame 3 {
                  }
                  frame 1, Default {
                    n695 = feedback #64(fxp<+,14,14> 0.0) -> (w1062:fxp<+,14,14>)
                    n696 = Add(x=w1059, y=w1062) -> (x+y=w1060:fxp<+,14,14>)
                    n697 = feedback-in #64(w1060) -> ()
                  }
                }
              }
              frame 2 {
                # "Changing increment of phase offset with each trap cycle. This results in a constant change in phase difference between trap cycles. \nOnly for traps 1 and 2 (set phase offset to zero for set three)."
                n698 = case shown="2" w1068 {
                  tunnel: w1067 -> [_ _ w1078]
                  tunnel: [w1069 fxp<+,14,14> 0.0 w1076] -> w1066
                  tunnel: w1064 -> [w1071 _ _]
                  tunnel: w1063 -> [w1072 _ w1079]
                  frame 2 {
                    n699 = Multiply(x=w1071, y=w1072) -> (x*y=w1070:fxp<+,16,16>)
                    n700 = feedback #65(fxp<+,14,14> 0.0) -> (w1074:fxp<+,14,14>)
                    n701 = Add(x=w1070, y=w1074) -> (x+y=w1069:fxp<+,14,14>)
                    n702 = feedback-in #65(w1069) -> ()
                  }
                  frame 3 {
                  }
                  frame 1, Default {
                    n703 = Multiply(x=w1078, y=w1079) -> (x*y=w1077:fxp<+,16,16>)
                    n704 = feedback #66(fxp<+,14,14> 0.0) -> (w1081:fxp<+,14,14>)
                    n705 = Add(x=w1077, y=w1081) -> (x+y=w1076:fxp<+,14,14>)
                    n706 = feedback-in #66(w1076) -> ()
                  }
                }
              }
              frame 3 {
                w1088 = u32 1013904223  # LCG constant C (add)
                w1090 = fxp<+,21,21> 1664525.0  # LCG constant A (multiply)
                # "Set a random phase offset. Random number generated using the LCG method. Constants and method taken from NI white noise generator code (method is general though)."
                # "shift to 14 significant bits"
                n707 = feedback #67(u32 4294967295 ("seed")) -> (w1085:u32)
                n708 = Multiply(x=w1085, y=w1090) -> (x*y=w1089:u32)
                n709 = Split Number(x=w1085) -> (hi(x)=w1091:u16)  [unwired: 1 out]
                n710 = To Unsigned Word Integer(number=w1091) -> (unsigned 16bit integer=w1083:u16)
                n711 = Add(x=w1089, y=w1088) -> (x+y=w1087:fxp<+,32,32>)
                n712 = To Unsigned Long Integer(number=w1087) -> (unsigned 32bit integer=w1084:u32)
                n713 = feedback-in #67(w1084) -> ()
                n714 = Scale By Power Of 2(n=i8 -2 ("Uniform scale factor"), x=w1083) -> (x*2^n=w1092:u16)
                n715 = To Fixed-Point(number=w1092) -> (fixed-point=w1082:fxp<+,14,14>)  [unwired: 1 in]
                "Random phase generated" <- w1082
                n716 = case shown="1, Default" w1096 {
                  tunnel: [w1097 fxp<+,14,14> 0.0 w1099] -> w1095
                  tunnel: w1082 -> [w1097 _ w1099]
                  frame 2 {
                  }
                  frame 3 {
                  }
                  frame 1, Default {
                  }
                }
              }
            }
            n717 = To Unsigned Word Integer(number=w949) -> (unsigned 16bit integer=w954:u16)
            n718 = Split Number(x=w954) -> (hi(x)=w952:u8, lo(x)=w953:u8)
            n719 = Split Number(x=u16 0) -> (hi(x)=w950:u8, lo(x)=w951:u8)
            n720 = Build Array ("BD 1 A Stack")(w952, w953) -> (w948:u8[])
            n721 = Build Array ("BD 1 A Stack")(w950, w951) -> (w947:u8[])
          }
        }
      }
    }
  }
  n722 = while "RF synth board interlacing timing loop" {
    tunnel: w2 -> [_]
    stop <- FALSE stop-if-true
    # "This loop is stalled until the RF FIFO get a value. With this method we gain additional delay time (because  we allow the rest of the main RF loop to procede while this loop waits to send the switch signals - a form of parallelism). This helps to simplify the main RF code. \n\nThe code also allow optimal interlacing while also controlling trap RF phase. \n\nNote: a lot of work has gone into optimizing these methods and it is unclear how they can be made any faster or better than this (many failed tries). Right now there is essentially ~4 ticks (~90 ns ns) of imperfection in the switching from trap 1 to trap 2. ~2 ticks of no RF (phase reset) then ~2 ticks of trap 2 with the wrong amplitude (T1 amplitude). The total ticks is 200, so not a big error.\n\nPhase can be precisely set for each trap. Phase reset and switching, has similar delays as fsk frequency switching. And phase reset and phase offset changes are also not simultaneous. So we can't perfectly line everything up.\n\nIf you start from amp zero though (as for trap 1), the on switch is perfect. Likewise the off is perfect for trap 2. \n\nThe green laser switching is also perfect because of its reduced duty cycle and delays in fsk switching between 80 and 0 MHz."
    n723 = xnode ("FIFO Read")("Timeout"=-1) -> ("Element"=w1505:u16, "FIFO Out"=w1501:refnum<k21>)  [unwired: 1 in, 1 out]
    n724 = Equal To 0?(x=w1505) -> (x = 0?=w1502:bool)
    n725 = Not(x=w1502) -> (.not. x?=w1459:bool)
    n726 = flat-sequence "BD 1 and 2 RF phase and amplitude switching" {
      tunnel: w1459 -> [_]
      tunnel: w1494 -> [w1609]
      tunnel: w1493 -> [w1608]
      tunnel: w1492 -> [w1607]
      tunnel: w1491 -> [w1606]
      tunnel: w1490 -> [w1605]
      tunnel: w1489 -> [w1604]
      tunnel: w1488 -> [w1603]
      tunnel: w1487 -> [w1602]
      tunnel: w1485 -> [w1601]
      tunnel: w1484 -> [w1600]
      tunnel: w1483 -> [w1599]
      tunnel: w1481 -> [w1597]
      tunnel: w1480 -> [w1596]
      tunnel: w1479 -> [w1595]
      tunnel: w1482 -> [w1598]
      tunnel: w1486 -> [w1594]
      tunnel: w1478 -> [w1633]
      tunnel: w1477 -> [w1632]
      tunnel: w1476 -> [w1631]
      tunnel: w1475 -> [w1630]
      tunnel: w1474 -> [w1629]
      tunnel: w1473 -> [w1628]
      tunnel: w1472 -> [w1627]
      tunnel: w1471 -> [w1626]
      tunnel: w1470 -> [w1625]
      tunnel: w1468 -> [w1624]
      tunnel: w1467 -> [w1623]
      tunnel: w1466 -> [w1622]
      tunnel: w1465 -> [w1621]
      tunnel: w1464 -> [w1620]
      tunnel: w1463 -> [w1619]
      tunnel: w1469 -> [w1618]
      frame #0 {
        # "Delay to align amp/frequency switching depending on the method used.\n\nCan also give enough time to do the parallel amplitude calculations"
        n727 = call "Wait"("Count(Ticks)"="Amp switch delay") -> ()  [unwired: 1 out]
      }
      frame #1 {
        w1589 = TRUE ("Connector1/DIO30")
        # "make phase offset and phase reset active with buffer transfer"
        n728 = xnode "FPGA I/O Node"("Connector1/DIO29"=w1589, "Connector1/DIO30"=w1589) -> ()  [unwired: 2 in, 2 out]
      }
      frame #2 {
        w1590 = FALSE ("Connector1/DIO15")
        # "write phase restart to buffer and reset udclk"
        n729 = xnode "FPGA I/O Node"("Connector1/DIO29"=w1590, "Connector1/DIO30"=w1590, "Connector1/DIO15"=FALSE ("Connector1/DIO14")) -> ()  [unwired: 3 in, 3 out]
      }
      frame #3 {
        w1592 = TRUE ("Connector1/DIO15")
        # "make phase restart active"
        # "reset WR"
        n730 = xnode "FPGA I/O Node"("Connector1/DIO15"=w1592, "Connector1/DIO29"=w1592, "Connector1/DIO30"=w1592) -> ()  [unwired: 3 in, 3 out]
      }
      frame #4 {
        w1593 = FALSE ("Connector1/DIO30")
        # "Address"
        # "set amp byte 1, and reset udclk"
        n731 = xnode "FPGA I/O Node"("Connector1/DIO0"=w1609, "Connector1/DIO1"=w1608, "Connector1/DIO2"=w1607, "Connector1/DIO3"=w1606, "Connector1/DIO4"=w1605, "Connector1/DIO5"=w1604, "Connector1/DIO6"=w1603, "Connector1/DIO7"=w1602, "Connector1/DIO8"=TRUE, "Connector1/DIO9"=FALSE, "Connector1/DIO10"=FALSE, "Connector1/DIO11"=FALSE, "Connector1/DIO12"=FALSE, "Connector1/DIO13"=TRUE, "Connector1/DIO20"=w1594, "Connector1/DIO21"=w1601, "Connector1/DIO22"=w1600, "Connector1/DIO23"=w1599, "Connector1/DIO24"=w1598, "Connector1/DIO25"=w1597, "Connector1/DIO26"=w1596, "Connector1/DIO27"=w1595, "Connector1/DIO30"=w1593, "Connector1/DIO29"=w1593) -> ()  [unwired: 24 in, 24 out]
      }
      frame #5 {
        # "write amp byte 1 to buffer"
        n732 = xnode "FPGA I/O Node"("Connector1/DIO15"=FALSE ("Connector1/DIO14")) -> ()  [unwired: 1 in, 1 out]
      }
      frame #6 {
        # "reset WR"
        n733 = xnode "FPGA I/O Node"("Connector1/DIO15"=TRUE) -> ()  [unwired: 1 in, 1 out]
      }
      frame #7 {
        # "Address"
        # "set amp byte 2"
        n734 = xnode "FPGA I/O Node"("Connector1/DIO0"=w1633, "Connector1/DIO1"=w1632, "Connector1/DIO2"=w1631, "Connector1/DIO3"=w1630, "Connector1/DIO4"=w1629, "Connector1/DIO5"=w1628, "Connector1/DIO6"=w1627, "Connector1/DIO7"=w1626, "Connector1/DIO8"=TRUE, "Connector1/DIO9"=FALSE, "Connector1/DIO10"=FALSE, "Connector1/DIO11"=FALSE, "Connector1/DIO12"=TRUE, "Connector1/DIO13"=FALSE, "Connector1/DIO20"=w1625, "Connector1/DIO21"=w1618, "Connector1/DIO22"=w1624, "Connector1/DIO23"=w1623, "Connector1/DIO24"=w1622, "Connector1/DIO25"=w1621, "Connector1/DIO26"=w1620, "Connector1/DIO27"=w1619) -> ()  [unwired: 22 in, 22 out]
      }
      frame #8 {
        # "write amp byte 2"
        n735 = xnode "FPGA I/O Node"("Connector1/DIO15"=FALSE ("Connector1/DIO14")) -> ()  [unwired: 1 in, 1 out]
      }
      frame #9 {
        w1641 = TRUE ("Connector1/DIO15")
        # "transfer amp bytes 1 and 2 and reset WR"
        n736 = xnode "FPGA I/O Node"("Connector1/DIO29"=w1641, "Connector1/DIO30"=w1641, "Connector1/DIO15"=TRUE ("Connector1/DIO14")) -> ()  [unwired: 3 in, 3 out]
      }
      frame #10 {
        w1643 = FALSE ("Connector1/DIO14")
        # "reset udclk"
        n737 = xnode "FPGA I/O Node"("Connector1/DIO29"=w1643, "Connector1/DIO30"=w1643) -> ()  [unwired: 2 in, 2 out]
      }
    }
    n738 = flat-sequence "FSK BD 1 (trap X)" {
      tunnel: w1459 -> [w1507]
      tunnel: [w1507] -> w1462
      tunnel: w1462 -> [w1508]
      frame #0 {
        n739 = call "Wait2"("Count(Ticks)"="BD 1 Delay (ticks)") -> ()  [unwired: 1 out]
      }
      frame #1 {
        # "switch frequency"
        n740 = xnode "FPGA I/O Node"("Connector1/DIO36"=w1508) -> ()  [unwired: 1 in, 1 out]
      }
    }
    n741 = flat-sequence "FSK BD 2 (trap Y or green laser AOM)" {
      tunnel: w1459 -> [w1645]
      tunnel: [w1645] -> w1504
      tunnel: w1504 -> [w1646]
      frame #0 {
        n742 = call "Wait11"("Count(Ticks)"="BD 2 Delay (Ticks)") -> ()  [unwired: 1 out]
      }
      frame #1 {
        # "switch frequency"
        n743 = xnode "FPGA I/O Node"("Connector1/DIO37"=w1646) -> ()  [unwired: 1 in, 1 out]
      }
    }
    n744 = xnode ("FIFO Read")("Timeout"=-1, "FIFO In"=w1501) -> ("Element"=w1496:u16, "FIFO Out"=w1500:refnum<k21>)  [unwired: 1 out]
    n745 = xnode ("FIFO Read")("Timeout"=-1, "FIFO In"=w1500) -> ("Element"=w1495:u16)  [unwired: 2 out]
    n746 = node-c288() -> (w1498:T6)  [unwired: 1 in]
    n747 = timed-loop "Convert amplitude words to bits" {
      timing: w1498 -> [_]
      timing-out: [_] -> w1497
      tunnel: w1496 -> [w1565]
      tunnel: w1495 -> [w1564]
      tunnel: [w1541] -> w1494
      tunnel: [w1540] -> w1493
      tunnel: [w1539] -> w1492
      tunnel: [w1538] -> w1491
      tunnel: [w1537] -> w1490
      tunnel: [w1536] -> w1489
      tunnel: [w1535] -> w1488
      tunnel: [w1534] -> w1487
      tunnel: [w1533] -> w1486
      tunnel: [w1532] -> w1485
      tunnel: [w1531] -> w1484
      tunnel: [w1530] -> w1483
      tunnel: [w1529] -> w1482
      tunnel: [w1528] -> w1481
      tunnel: [w1527] -> w1480
      tunnel: [w1526] -> w1479
      tunnel: [w1525] -> w1478
      tunnel: [w1524] -> w1477
      tunnel: [w1523] -> w1476
      tunnel: [w1522] -> w1475
      tunnel: [w1521] -> w1474
      tunnel: [w1520] -> w1473
      tunnel: [w1519] -> w1472
      tunnel: [w1518] -> w1471
      tunnel: [w1517] -> w1470
      tunnel: [w1516] -> w1469
      tunnel: [w1515] -> w1468
      tunnel: [w1514] -> w1467
      tunnel: [w1513] -> w1466
      tunnel: [w1512] -> w1465
      tunnel: [w1511] -> w1464
      tunnel: [w1510] -> w1463
      stop <- TRUE stop-if-true
      # "Board 1 Data"
      # "Board 2 Data"
      # "Board 1 Data"
      # "Board 2 Data"
      n748 = Split Number(x=w1565) -> (hi(x)=w1563:u8, lo(x)=w1543:u8)
      n749 = Split Number(x=w1564) -> (hi(x)=w1562:u8, lo(x)=w1542:u8)
      n750 = Number To Boolean Array(number=w1563) -> (Boolean array=w1583:bool[])
      n751 = Number To Boolean Array(number=w1562) -> (Boolean array=w1574:bool[])
      n752 = Index Array(array=w1583, index=7) -> (element=w1541:bool)
      n753 = Index Array(array=w1583, index=6) -> (element=w1540:bool)
      n754 = Index Array(array=w1583, index=5) -> (element=w1539:bool)
      n755 = Index Array(array=w1583, index=4) -> (element=w1538:bool)
      n756 = Index Array(array=w1583, index=3) -> (element=w1537:bool)
      n757 = Index Array(array=w1583, index=2) -> (element=w1536:bool)
      n758 = Index Array(array=w1583, index=1) -> (element=w1535:bool)
      n759 = Index Array(array=w1583, index=0) -> (element=w1534:bool)
      n760 = Index Array(array=w1574, index=7) -> (element=w1533:bool)
      n761 = Index Array(array=w1574, index=6) -> (element=w1532:bool)
      n762 = Index Array(array=w1574, index=5) -> (element=w1531:bool)
      n763 = Index Array(array=w1574, index=4) -> (element=w1530:bool)
      n764 = Index Array(array=w1574, index=3) -> (element=w1529:bool)
      n765 = Index Array(array=w1574, index=2) -> (element=w1528:bool)
      n766 = Index Array(array=w1574, index=1) -> (element=w1527:bool)
      n767 = Index Array(array=w1574, index=0) -> (element=w1526:bool)
      n768 = Number To Boolean Array(number=w1543) -> (Boolean array=w1561:bool[])
      n769 = Number To Boolean Array(number=w1542) -> (Boolean array=w1552:bool[])
      n770 = Index Array(array=w1561, index=7) -> (element=w1525:bool)
      n771 = Index Array(array=w1561, index=6) -> (element=w1524:bool)
      n772 = Index Array(array=w1561, index=5) -> (element=w1523:bool)
      n773 = Index Array(array=w1561, index=4) -> (element=w1522:bool)
      n774 = Index Array(array=w1561, index=3) -> (element=w1521:bool)
      n775 = Index Array(array=w1561, index=2) -> (element=w1520:bool)
      n776 = Index Array(array=w1561, index=1) -> (element=w1519:bool)
      n777 = Index Array(array=w1561, index=0) -> (element=w1518:bool)
      n778 = Index Array(array=w1552, index=7) -> (element=w1517:bool)
      n779 = Index Array(array=w1552, index=6) -> (element=w1516:bool)
      n780 = Index Array(array=w1552, index=5) -> (element=w1515:bool)
      n781 = Index Array(array=w1552, index=4) -> (element=w1514:bool)
      n782 = Index Array(array=w1552, index=3) -> (element=w1513:bool)
      n783 = Index Array(array=w1552, index=2) -> (element=w1512:bool)
      n784 = Index Array(array=w1552, index=1) -> (element=w1511:bool)
      n785 = Index Array(array=w1552, index=0) -> (element=w1510:bool)
    }
    n786 = node-c288(w1497) -> ()
  }
  n787 = while "Control APD data integration - stream to host" {
    shift-right: [w1650] -> _
    shift-left: w1 -> [w1655]
    stop <- FALSE stop-if-true
    n788 = flat-sequence {
      tunnel: w1655 -> [w1657]
      tunnel: [w1658] -> w1653
      tunnel: [w1657] -> w1651
      tunnel: [w1668] -> w1654
      tunnel: w1653 -> [w1668]
      tunnel: [w1667] -> w1652
      tunnel: w1651 -> [w1667]
      tunnel: [w1666] -> w1649
      tunnel: [w1665] -> w1648
      tunnel: [w1659] -> w1647
      tunnel: [w1716] -> w1650
      tunnel: w1654 -> [w1725]
      tunnel: w1652 -> [w1722]
      tunnel: w1649 -> [w1709]
      tunnel: w1648 -> [w1708]
      tunnel: w1647 -> [w1696]
      frame #0 {
        n789 = call "Loop Timer6"("Count(Ticks)"=w1657) -> ("Tick Count(Ticks)"=w1658:u32)
      }
      frame #1 {
        n790 = flat-sequence {
          tunnel: [w1670] -> w1664
          tunnel: w1664 -> [w1674]
          tunnel: [w1676] -> w1663
          tunnel: [w1675] -> w1662
          tunnel: [w1674] -> w1661
          tunnel: [i16 0] -> w1660
          tunnel: [w1687] -> w1665
          tunnel: [w1688] -> w1666
          tunnel: w1663 -> [w1688]
          tunnel: w1662 -> [w1687]
          tunnel: w1661 -> [w1686]
          tunnel: w1660 -> [w1685]
          tunnel: [w1685] -> w1659
          frame #0 {
            # "use separate variable so each APD won't\nhave to wait to read"
            n791 = feedback #68(FALSE) -> (w1669:bool)
            "APD1 out state" <- w1669
            "APD2 out state" <- w1669
            n792 = disable-structure shown="Disabled" {
              disable-tunnel: w1669 -> [w1672 _]
              frame Disabled {
                "APD3 out state" <- w1672
              }
              frame Enabled {
              }
            }
            n793 = Not(x=w1669) -> (.not. x?=w1670:bool)
            n794 = feedback-in #68(w1670) -> ()
          }
          frame #1 {
            n795 = disable-structure shown="Disabled" {
              disable-tunnel: w1674 -> [w1682 _]
              disable-tunnel: [w1681 _] -> _
              frame Disabled {
                n796 = local read "APD 3 Counts 1"() -> (w1684:u32)
                n797 = local read "APD 3 Counts 0"() -> (w1683:u32)
                n798 = Select(t=w1684, s=w1682, f=w1683) -> (s? t:f=w1681:u32)
              }
              frame Enabled {
              }
            }
            n799 = local read "APD 1 Counts 1"() -> (w1680:u32)
            n800 = local read "APD 1 Counts 0"() -> (w1679:u32)
            n801 = local read "APD 2 Counts 1"() -> (w1678:u32)
            n802 = local read "APD 2 Counts 0"() -> (w1677:u32)
            n803 = Select(t=w1680, s=w1674, f=w1679) -> (s? t:f=w1676:u32)
            n804 = Select(t=w1678, s=w1674, f=w1677) -> (s? t:f=w1675:u32)
          }
          frame #2 {
            n805 = case shown="True" w1686 {
              frame False {
                w1689 = u32 0 ("APD 1 Counts 0")
                n806 = disable-structure shown="Disabled" {
                  disable-tunnel: w1689 -> [w1690 _]
                  frame Disabled {
                    n807 = local write "APD 3 Counts 0"(w1690) -> ()
                  }
                  frame Enabled {
                  }
                }
                n808 = local write "APD 1 Counts 0"(w1689) -> ()
                n809 = local write "APD 2 Counts 0"(w1689) -> ()
              }
              frame True {
                w1691 = u32 0 ("APD 1 Counts 1")
                n810 = disable-structure shown="Disabled" {
                  disable-tunnel: w1691 -> [w1692 _]
                  frame Disabled {
                    n811 = local write "APD 3 Counts 1"(w1692) -> ()
                  }
                  frame Enabled {
                  }
                }
                n812 = local write "APD 1 Counts 1"(w1691) -> ()
                n813 = local write "APD 2 Counts 1"(w1691) -> ()
              }
            }
          }
        }
      }
      frame #2 {
        # "crude initialization: if APD to FIFO is off (usually\nonly before initializing a measurement) count is forced to 0\nand green to true"
        # "count cycles till switching"
        n814 = feedback-in #69(w1725) -> ()
        n815 = feedback #69(w1725) -> (w1724:u32)
        n816 = Subtract(x=w1725, y=w1724) -> (x-y=w1723:u32)
        n817 = Subtract(x=w1723, y=w1722) -> (x-y=w1701:u32)
        n818 = case shown="True" "APD to FIFO" {
          tunnel: w1709 -> [_ w1730]
          tunnel: w1708 -> [_ w1728]
          tunnel: w1696 -> [_ w1726]
          frame False {
          }
          frame True {
            n819 = flat-sequence {
              tunnel: 0 ("Timeout") -> [w1732]
              tunnel: w1730 -> [w1733]
              tunnel: [w1732] -> w1729
              tunnel: w1729 -> [w1734]
              tunnel: w1728 -> [w1735]
              tunnel: [w1734] -> w1727
              tunnel: w1727 -> [w1737]
              tunnel: w1726 -> [w1736]
              frame #0 {
                n820 = xnode ("FIFO Write")("Element"=w1733, "Timeout"=w1732) -> ()  [unwired: 1 in, 2 out]
              }
              frame #1 {
                n821 = xnode ("FIFO Write")("Element"=w1735, "Timeout"=w1734) -> ()  [unwired: 1 in, 2 out]
              }
              frame #2 {
                n822 = xnode ("FIFO Write")("Element"=w1736, "Timeout"=w1737) -> ()  [unwired: 1 in, 2 out]
              }
            }
          }
        }
        n823 = Subtract(x="APD Acq Rate Count", y=w1701) -> (x-y=w1717:u32)
        n824 = Number To Boolean Array(number=w1701) -> (Boolean array=w1702:bool[])
        n825 = Or Array Elements(Boolean array=w1702) -> (logical OR=w1700:bool)
        n826 = Boolean To (0,1)(Boolean=w1700) -> (0, 1=w1707:i16)
        n827 = To Unsigned Byte Integer(number=w1707) -> (unsigned 8bit integer=w1704:u8)
        n828 = feedback #70(u8 0) -> (w1705:u8)
        n829 = Add(x=w1704, y=w1705) -> (x+y=w1703:u8)
        "APD Acq Late Counter" <- w1703
        n830 = feedback-in #70(w1703) -> ()
        n831 = Boolean To (0,1)(Boolean="+ phase (APD Acq)") -> (0, 1=w1713:i16)
        n832 = Multiply(x=w1713, y="Phase Count Adjustment (APD Acq)") -> (x*y=w1710:i16)
        n833 = Add(x=w1717, y=w1710) -> (x+y=w1716:u32)
        n834 = feedback #71(i16 0) -> (w1715:i16)
        n835 = Subtract(x=w1715, y=w1710) -> (x-y=w1712:i16)
        "APD Acq Relative Phase" <- w1712
        n836 = feedback-in #71(w1712) -> ()
        n837 = To Word Integer(number=w1709) -> (16bit integer=w1718:i16)
        n838 = To Word Integer(number=w1696) -> (16bit integer=w1697:i16)
        n839 = To Word Integer(number=w1708) -> (16bit integer=w1719:i16)
        n840 = Multiply(x="APD AO scale factor", y=w1719) -> (x*y=w1698:i16)
        n841 = Multiply(x="APD AO scale factor", y=w1697) -> (x*y=w1694:i16)
        n842 = Multiply(x="APD AO scale factor", y=w1718) -> (x*y=w1699:i16)
        n843 = xnode "FPGA I/O Node"("Connector0/AO5"=w1699, "Connector0/AO7"=w1698, "Connector0/AO6"=w1694) -> ()  [unwired: 3 in, 3 out]
      }
    }
  }
  n844 = disable-structure shown="Disabled" {
    disable-tunnel: w2 -> [w1738 _]
    frame Disabled {
      n845 = while "APD 3 Counter" {
        tunnel: w1738 -> [_]
        stop <- FALSE stop-if-true
        n846 = flat-sequence {
          frame #0 {
            n847 = xnode "FPGA I/O Method Node"("FPGA I/O In"=refnum<k21> "Connector0/DIO12" ("APD 2 DO"), "Timeout"=-1) -> ()  [unwired: 2 out]
          }
          frame #1 {
            n848 = local read "APD3 int gate"() -> (w1742:bool)
            n849 = case shown="True" w1742 {
              frame False {
              }
              frame True {
                n850 = local read "APD3 out state"() -> (w1743:bool)
                n851 = case shown="True" w1743 {
                  frame False {
                    n852 = local read "APD 3 Counts 0"() -> (w1745:u32)
                    n853 = Increment(x=w1745) -> (x+1=→"APD 3 Counts 0":u32)
                  }
                  frame True {
                    n854 = local read "APD 3 Counts 1"() -> (w1747:u32)
                    n855 = Increment(x=w1747) -> (x+1=→"APD 3 Counts 1":u32)
                  }
                }
              }
            }
          }
        }
      }
    }
    frame Enabled {
    }
  }
  n856 = disable-structure shown="Disabled" {
    disable-tunnel: w2 -> [w1749 _]
    disable-tunnel: w3 -> [w1748 _]
    frame Disabled {
      n857 = while "APD 3 Gating" {
        shift-right: [w1753] -> _
        shift-left: w1749 -> [w1758]
        shift-right: [w1752] -> _
        shift-left: w1748 -> [w1750]
        stop <- FALSE stop-if-true
        n858 = flat-sequence {
          tunnel: w1758 -> [w1761]
          tunnel: [w1762] -> w1756
          tunnel: [w1761] -> w1754
          tunnel: [w1760] -> w1751
          tunnel: w1750 -> [w1760]
          tunnel: [w1765] -> w1757
          tunnel: w1756 -> [w1765]
          tunnel: [w1764] -> w1755
          tunnel: w1754 -> [w1764]
          tunnel: w1751 -> [w1763]
          tunnel: [w1786] -> w1753
          tunnel: w1757 -> [w1797]
          tunnel: w1755 -> [w1794]
          tunnel: [w1766] -> w1752
          frame #0 {
            n859 = call "Loop Timer15"("Count(Ticks)"=w1761) -> ("Tick Count(Ticks)"=w1762:u16)
          }
          frame #1 {
            # "Signal maybe then sent through \na transistor before APD"
            n860 = xnode "FPGA I/O Node"("Connector0/DIO2"=w1763) -> ()  [unwired: 1 in, 1 out]
            "APD3 int gate" <- w1763
          }
          frame #2 {
            n861 = local read "APD Gate OFF Count"() -> (w1771:u16)
            n862 = local read "APD Gate ON Count"() -> (w1772:u16)
            n863 = feedback #72(TRUE) -> (w1791:bool)
            n864 = feedback-in #73(w1797) -> ()
            n865 = feedback #73(w1797) -> (w1796:u16)
            n866 = Not(x=w1791) -> (.not. x?=w1789:bool)
            n867 = feedback-in #72(w1789) -> ()
            n868 = Subtract(x=w1797, y=w1796) -> (x-y=w1795:u16)
            n869 = Select(t=w1772, s=w1789, f=w1771) -> (s? t:f=w1793:u16)
            n870 = Subtract(x=w1795, y=w1794) -> (x-y=w1774:u16)
            n871 = Subtract(x=w1793, y=w1774) -> (x-y=w1785:u16)
            n872 = Number To Boolean Array(number=w1774) -> (Boolean array=w1775:bool[])
            n873 = Or Array Elements(Boolean array=w1775) -> (logical OR=w1773:bool)
            n874 = Boolean To (0,1)(Boolean=w1773) -> (0, 1=w1780:i16)
            n875 = Boolean To (0,1)(Boolean="+ phase (APD 3 Gate)") -> (0, 1=w1783:i16)
            n876 = To Unsigned Byte Integer(number=w1780) -> (unsigned 8bit integer=w1777:u8)
            n877 = Multiply(x=w1783, y="Phase count adjustment (APD 3 Gate)") -> (x*y=w1781:i16)
            n878 = feedback #74(u8 0) -> (w1778:u8)
            n879 = Add(x=w1777, y=w1778) -> (x+y=w1776:u8)
            "APD 3 Gate Late Counter" <- w1776
            n880 = feedback-in #74(w1776) -> ()
            n881 = Add(x=w1785, y=w1781) -> (x+y=w1786:u16)
            n882 = feedback #75(i16 0) -> (w1788:i16)
            n883 = Subtract(x=w1788, y=w1781) -> (x-y=w1787:i16)
            "APD 3 Gate Relative Phase" <- w1787
            n884 = feedback-in #75(w1787) -> ()
            n885 = local read "APD Gate Operating Mode"() -> (w1770:u8)
            n886 = case shown="2" w1770 {
              tunnel: [TRUE FALSE w1800] -> w1767
              tunnel: w1791 -> [_ _ w1800]
              frame 0, Default {
              }
              frame 1 {
              }
              frame 2 {
              }
            }
            n887 = local read "Invert APD Gate"() -> (w1769:bool)
            n888 = Not(x=w1767) -> (.not. x?=w1768:bool)
            n889 = Select(t=w1768, s=w1769, f=w1767) -> (s? t:f=w1766:bool)
          }
        }
      }
    }
    frame Enabled {
    }
  }
  n890 = while {
    shift-right: [w1803] -> _
    shift-left: w2 -> [w1809]
    shift-right: [w1804] -> _
    shift-left: _ -> [w1801]
    stop <- FALSE stop-if-true
    n891 = flat-sequence {
      tunnel: w1809 -> [w1812]
      tunnel: [w1813] -> w1807
      tunnel: [w1812] -> w1805
      tunnel: [w1811] -> w1802
      tunnel: w1801 -> [w1811]
      tunnel: [w1816] -> w1808
      tunnel: w1807 -> [w1816]
      tunnel: [w1815] -> w1806
      tunnel: w1805 -> [w1815]
      tunnel: w1802 -> [w1814]
      tunnel: w1808 -> [w1846]
      tunnel: w1806 -> [w1845]
      tunnel: [w1818] -> w1804
      tunnel: [w1817] -> w1803
      frame #0 {
        n892 = call "Loop Timer2"("Count(Ticks)"=w1812) -> ("Tick Count(Ticks)"=w1813:u16)
      }
      frame #1 {
        n893 = xnode "FPGA I/O Node"("Connector0/DIO10"=w1814) -> ()  [unwired: 1 in, 1 out]
      }
      frame #2 {
        n894 = feedback #76(w1846) -> (w1847:u16)
        n895 = feedback-in #76(w1846) -> ()
        n896 = Subtract(x=w1846, y=w1847) -> (x-y=w1848:u16)
        n897 = Subtract(x=w1848, y=w1845) -> (x-y=w1838:u16)
        n898 = Number To Boolean Array(number=w1838) -> (Boolean array=w1843:bool[])
        n899 = Or Array Elements(Boolean array=w1843) -> (logical OR=w1844:bool)
        n900 = Boolean To (0,1)(Boolean="+ phase (EMCCD Gate)") -> (0, 1=w1831:i16)
        n901 = Boolean To (0,1)(Boolean=w1844) -> (0, 1=w1839:i16)
        n902 = To Unsigned Byte Integer(number=w1839) -> (unsigned 8bit integer=w1842:u8)
        n903 = Multiply(x=w1831, y="Phase Count Adjustment EMCCD Gate") -> (x*y=w1833:i16)
        n904 = feedback #77(u8 0) -> (w1841:u8)
        n905 = Add(x=w1842, y=w1841) -> (x+y=w1837:u8)
        "EMCCD Late counter" <- w1837
        n906 = feedback-in #77(w1837) -> ()
        n907 = feedback #78(i16 0) -> (w1832:i16)
        n908 = Subtract(x=w1832, y=w1833) -> (x-y=w1826:i16)
        "EMCCD relative phase" <- w1826
        n909 = feedback-in #78(w1826) -> ()
        n910 = feedback #79(TRUE) -> (w1824:bool)
        n911 = Not(x=w1824) -> (.not. x?=w1822:bool)
        n912 = Select(t="EMCCD Gate ON count", s=w1822, f="EMCCD Gate OFF count") -> (s? t:f=w1834:u16)
        n913 = Subtract(x=w1834, y=w1838) -> (x-y=w1827:u16)
        n914 = Add(x=w1827, y=w1833) -> (x+y=w1817:u16)
        n915 = feedback-in #79(w1822) -> ()
        n916 = case shown="1" "EMCCD Gate Operating Mode" {
          tunnel: w1822 -> [_ _ w1851]
          tunnel: [TRUE FALSE w1851] -> w1820
          frame 0, Default {
          }
          frame 1 {
          }
          frame 2 {
          }
        }
        n917 = Not(x=w1820) -> (.not. x?=w1821:bool)
        n918 = Select(t=w1821, s="Invert EMCCD Gate", f=w1820) -> (s? t:f=w1818:bool)
      }
    }
  }
  n919 = disable-structure shown="Disabled" {
    disable-tunnel: w2 -> [w1854 _]
    disable-tunnel: w14 -> [w1853 _]
    frame Disabled {
      n920 = while "633 nm red  fluorescent laser interlacing (DO to IA 633 nm AOM ME amp)." {
        shift-right: [w1975] -> _
        shift-left: w1854 -> [w1980]
        shift-right: [w1974] -> _
        shift-left: w1853 -> [w1972]
        stop <- FALSE stop-if-true
        n921 = flat-sequence {
          tunnel: w1980 -> [w1983]
          tunnel: [w1984] -> w1978
          tunnel: [w1983] -> w1976
          tunnel: [w1982] -> w1973
          tunnel: w1972 -> [w1982]
          tunnel: [w1987] -> w1979
          tunnel: w1978 -> [w1987]
          tunnel: [w1986] -> w1977
          tunnel: w1976 -> [w1986]
          tunnel: w1973 -> [w1985]
          tunnel: [w1996] -> w1975
          tunnel: w1979 -> [w2016]
          tunnel: w1977 -> [w2013]
          tunnel: [w2005] -> w1974
          frame #0 {
            n922 = call "Loop Timer11"("Count(Ticks)"=w1983) -> ("Tick Count(Ticks)"=w1984:u16)
          }
          frame #1 {
            # "Then to PRL 440 amp"
            n923 = xnode "FPGA I/O Node"("Connector1/DIO32"=w1985) -> ()  [unwired: 1 in, 1 out]
          }
          frame #2 {
            n924 = feedback-in #80(w2016) -> ()
            n925 = feedback #80(w2016) -> (w2015:u16)
            n926 = Subtract(x=w2016, y=w2015) -> (x-y=w2014:u16)
            n927 = Subtract(x=w2014, y=w2013) -> (x-y=w1989:u16)
            n928 = Number To Boolean Array(number=w1989) -> (Boolean array=w1990:bool[])
            n929 = Or Array Elements(Boolean array=w1990) -> (logical OR=w1988:bool)
            n930 = Boolean To (0,1)(Boolean="+ phase (RI)") -> (0, 1=w2001:i16)
            n931 = Multiply(x=w2001, y="Phase count adjustment (RI)") -> (x*y=w1998:i16)
            n932 = Boolean To (0,1)(Boolean=w1988) -> (0, 1=w1995:i16)
            n933 = To Unsigned Byte Integer(number=w1995) -> (unsigned 8bit integer=w1992:u8)
            n934 = feedback #81(i16 0) -> (w1999:i16)
            n935 = feedback #82(u8 0) -> (w1993:u8)
            n936 = Add(x=w1992, y=w1993) -> (x+y=w1991:u8)
            "RI Late Counter" <- w1991
            n937 = feedback-in #82(w1991) -> ()
            n938 = Subtract(x=w1999, y=w1998) -> (x-y=w1997:i16)
            "RI Relative phase" <- w1997
            n939 = feedback-in #81(w1997) -> ()
            n940 = feedback #83(TRUE) -> (w2008:bool)
            n941 = case shown="2" "Red Laser Operating Mode" {
              tunnel: [TRUE FALSE w2022] -> w2005
              tunnel: w2008 -> [_ _ w2019]
              frame 0, Default {
              }
              frame 1 {
              }
              frame 2 {
                n942 = Not(x=w2019) -> (.not. x?=w2021:bool)
                n943 = Select(t=w2021, s="Invert RI", f=w2019) -> (s? t:f=w2022:bool)
              }
            }
            n944 = Not(x=w2008) -> (.not. x?=w2004:bool)
            n945 = Select(t="Red interlace ON count", s=w2004, f="Red interlace OFF count") -> (s? t:f=w2010:u16)
            n946 = Subtract(x=w2010, y=w1989) -> (x-y=w2002:u16)
            n947 = Add(x=w2002, y=w1998) -> (x+y=w1996:u16)
            n948 = feedback-in #83(w2004) -> ()
          }
        }
      }
      n949 = while "473 nm blue  fluorescent laser interlacing (DO to blue laser digital control input)." {
        shift-right: [w1871] -> _
        shift-left: w1854 -> [w1874]
        shift-right: [w1870] -> _
        shift-left: w1853 -> [w1868]
        shift-right: [w1863] -> _
        shift-left: _ -> [w1862]
        shift-right: [w1855] -> _
        shift-left: u16 0 -> [w1858]
        stop <- FALSE stop-if-true
        n950 = flat-sequence {
          tunnel: w1874 -> [w1879]
          tunnel: [w1880] -> w1873
          tunnel: [w1879] -> w1872
          tunnel: [w1878] -> w1869
          tunnel: w1868 -> [w1878]
          tunnel: w1862 -> [w1877]
          tunnel: [w1877] -> w1861
          tunnel: [w1876] -> w1859
          tunnel: w1858 -> [w1876]
          tunnel: [w1885] -> w1867
          tunnel: w1873 -> [w1885]
          tunnel: [w1884] -> w1866
          tunnel: w1872 -> [w1884]
          tunnel: w1869 -> [w1883]
          tunnel: w1861 -> [w1882]
          tunnel: [w1882] -> w1860
          tunnel: w1859 -> [w1881]
          tunnel: [w1881] -> w1857
          tunnel: [w1890] -> w1865
          tunnel: [w1889] -> w1864
          tunnel: w1866 -> [w1889]
          tunnel: w1867 -> [w1890]
          tunnel: w1860 -> [w1888]
          tunnel: w1857 -> [w1887]
          tunnel: [w1886] -> w1856
          tunnel: [w1947] -> w1871
          tunnel: w1865 -> [w1965]
          tunnel: w1864 -> [w1962]
          tunnel: [w1935] -> w1870
          tunnel: [w1933] -> w1863
          tunnel: w1856 -> [w1930]
          tunnel: [w1931] -> w1855
          frame #0 {
            n951 = call "Loop Timer14"("Count(Ticks)"=w1879) -> ("Tick Count(Ticks)"=w1880:u16)
          }
          frame #1 {
            n952 = xnode "FPGA I/O Node"("Connector1/DIO28"=w1883) -> ()  [unwired: 1 in, 1 out]
          }
          frame #2 {
            n953 = case shown="True" w1888 {
              tunnel: w1887 -> [w1891 w1893]
              tunnel: [w1891 w1892] -> w1886
              frame False {
              }
              frame True {
                n954 = flat-sequence {
                  tunnel: [w1899] -> w1896
                  tunnel: [w1898] -> w1895
                  tunnel: [w1897] -> w1894
                  tunnel: w1893 -> [w1897]
                  tunnel: w1896 -> [w1916]
                  tunnel: w1895 -> [w1913]
                  tunnel: w1894 -> [w1915]
                  tunnel: [w1914] -> w1892
                  frame #0 {
                    # "5 ns timing resolution"
                    n955 = node-c288() -> (w1902:T6)  [unwired: 1 in]
                    n956 = timed-loop {
                      timing: w1902 -> [_]
                      timing-out: [_] -> w1901
                      tunnel: "Lifetime timeout APD1" -> [w1908]
                      tunnel: [w1903] -> w1898
                      tunnel: [w1904] -> w1899
                      i -> [w1905]
                      stop <- w1907 stop-if-true
                      n957 = xnode "FPGA I/O Node"() -> ("Connector0/DIO5"=w1906:bool)  [unwired: 1 in, 1 out]
                      n958 = To Unsigned Word Integer(number=w1905) -> (unsigned 16bit integer=w1903:u16)
                      n959 = Equal?(x=w1908, y=w1903) -> (x = y?=w1904:bool)
                      n960 = Or(x=w1906, y=w1904) -> (x .or. y?=w1907:bool)
                    }
                    n961 = node-c288(w1901) -> ()
                  }
                  frame #1 {
                    n962 = Not(x=w1916) -> (.not. x?=w1917:bool)
                    n963 = case shown="True" w1917 {
                      tunnel: w1913 -> [_ w1919]
                      tunnel: w1915 -> [w1918 w1921]
                      tunnel: [w1918 w1920] -> w1914
                      frame False {
                        # "timed out, do nothing"
                      }
                      frame True {
                        # "photon detected,record time"
                        n964 = case shown="True" "Lifetime to FIFO" {
                          tunnel: w1919 -> [_ w1927]
                          tunnel: w1921 -> [w1923 w1925]
                          tunnel: [w1923 w1924] -> w1920
                          frame False {
                            # "don't record time\n(can't if doing force feedback)"
                          }
                          frame True {
                            # "number of events in fifo"
                            n965 = xnode ("FIFO Method Node")("Element"=w1927, "Timeout"=0) -> ()  [unwired: 1 in, 2 out]
                            n966 = Increment(x=w1925) -> (x+1=w1924:u16)
                          }
                        }
                        "lifetime (ticks)" <- w1919
                      }
                    }
                  }
                }
              }
            }
          }
          frame #3 {
            # "Reading fifo is tricky here since\nunknown # of events"
            # "For lifetime measurement:\nInterlacing and pulse falling"
            n967 = feedback-in #84(w1965) -> ()
            n968 = feedback #84(w1965) -> (w1964:u16)
            n969 = Subtract(x=w1965, y=w1964) -> (x-y=w1963:u16)
            n970 = Subtract(x=w1963, y=w1962) -> (x-y=w1940:u16)
            n971 = Number To Boolean Array(number=w1940) -> (Boolean array=w1941:bool[])
            n972 = Or Array Elements(Boolean array=w1941) -> (logical OR=w1939:bool)
            n973 = Boolean To (0,1)(Boolean="+ phase (BI D)") -> (0, 1=w1952:i16)
            n974 = Multiply(x=w1952, y="Phase count adjustment (BI D)") -> (x*y=w1949:i16)
            n975 = Boolean To (0,1)(Boolean=w1939) -> (0, 1=w1946:i16)
            n976 = To Unsigned Byte Integer(number=w1946) -> (unsigned 8bit integer=w1943:u8)
            n977 = feedback #85(i16 0) -> (w1950:i16)
            n978 = feedback #86(u8 0) -> (w1944:u8)
            n979 = Add(x=w1943, y=w1944) -> (x+y=w1942:u8)
            "Blue Late Counter (D)" <- w1942
            n980 = feedback-in #86(w1942) -> ()
            n981 = Subtract(x=w1950, y=w1949) -> (x-y=w1948:i16)
            "BI Relative phase (D)" <- w1948
            n982 = feedback-in #85(w1948) -> ()
            n983 = feedback #87(TRUE) -> (w1957:bool)
            n984 = case shown="2" "Blue Laser Operating Mode (D)" {
              tunnel: [TRUE FALSE w1971] -> w1935
              tunnel: w1957 -> [_ _ w1968]
              frame 0, Default {
              }
              frame 1 {
              }
              frame 2 {
                n985 = Not(x=w1968) -> (.not. x?=w1970:bool)
                n986 = Select(t=w1970, s="Invert BI (D)", f=w1968) -> (s? t:f=w1971:bool)
              }
            }
            n987 = Subtract(x=w1930, y="Lifetime events to read blue") -> (x-y=w1928:u16)
            n988 = Not(x=w1957) -> (.not. x?=w1955:bool)
            n989 = Select(t="Blue interlace ON count (D)", s=w1955, f="Blue interlace OFF count (D)") -> (s? t:f=w1959:u16)
            n990 = Subtract(x=w1959, y=w1940) -> (x-y=w1953:u16)
            n991 = Add(x=w1953, y=w1949) -> (x+y=w1947:u16)
            n992 = feedback-in #87(w1955) -> ()
            n993 = Select(t=w1928, s="Lifetime read blue fifo", f=w1930) -> (s? t:f=w1931:u16)
            "lifetime events in fifo" <- w1931
            n994 = Equal?(x="Blue Laser Operating Mode (D)", y=u8 2) -> (x = y?=w1936:bool)
            n995 = Not(x=w1935) -> (.not. x?=w1934:bool)
            n996 = And(x=w1934, y=w1936) -> (x .and. y?=w1933:bool)
          }
        }
      }
    }
    frame Enabled {
    }
  }
